vi "host 1st.vi"() -> ()   [LabVIEW 2017]
uses:
  b7b9a1d8-5f4e-4797-a25c-3bdebfd9df9c.vi
  globals/Global variables.vi
  globals/RIO and DAC defaults global.vi
  globals/Modules global.vi
  globals/DIO board parameters global.vi
  <vilib>/FPGAPlugInAG/PXI-7811R/niLvFpga_Open_PXI-7811R.vi
  <vilib>/rvi/interface/common/dynamic/niFpgaDynamicAddResources.vi
  <vilib>/rvi/interface/nirviOpenFPGA/nirviOpenFPGA.xnode
  FPGA Bitfiles/project1_FPGATarget_statemachine_BoC7x3TXtqU.lvbitx
  FPGA vi/state machine.vi
panel:
  out "GPIB output":T1(array[cluster])=[{"Enable"=TRUE, "Abs Start Time"=26343.857, "Module"=31, "String"="FREQ 2 MHz;", "Array"=["27", ""]}, {"Enable"=TRUE, "Abs Start Time"=27143.857, "Module"=31, "String"="ENBR 1;", "Array"=["27", ""]}, {"Enable"=TRUE, "Abs Start Time"=29143.857, "Module"=31, "String"="ENBR 0;", "Array"=["27", ""]}]
  out "AO indicator 3":dbl[][](array[numeric])
  in  "DAC timeline enables 3":bool[](array[boolean])=[FALSE, FALSE, FALSE, FALSE, FALSE, FALSE, FALSE, TRUE]
  out "DAC timelines 3":T2(graph)=[{"times"=[], "Static DAC Array"=[]}, {"times"=[], "Static DAC Array"=[]}, {"times"=[], "Static DAC Array"=[]}, {"times"=[], "Static DAC Array"=[]}, {"times"=[], "Static DAC Array"=[]}, {"times"=[], "Static DAC Array"=[]}, {"times"=[], "Static DAC Array"=[]}, {"times"=[0.1, 1501.0, 1501.1, 1501.2, 1501.3, 1501.4, 1501.5, 1501.6, 1501.7, 1501.8, 1501.9, 1502.0, 1600.0, 1700.0, 1800.0, 8000.0], "Static DAC Array"=[0.0, 0.0, 0.5, 1.0, 1.5, 2.0, 2.5, 3.0, 3.5, 4.0, 4.5, 5.0, 1.0, 2.0, 3.0, 0.0]}]
  in  "DAC force enables 3":bool[](array[boolean])=[FALSE, FALSE, FALSE, FALSE, FALSE, FALSE, FALSE, FALSE]
  in  "DAC force volts 3":dbl[](array[numeric])=[0.0, 0.0, 0.0, 0.0, 0.0, 0.0, 0.0, 0.0]
  out "DAC channel discription 3":string[](array[string])=["", "", "", "", "", "", "", "\n"]
  out "number 2":ext=24208.27054977417 format="%#_9g"
  out "number":ext=2000.0 format="%#_9g"
  out "Boolean 6":bool
  out "Boolean 5":bool
  out "Boolean 4":bool
  out "Boolean 3":bool
  out "Boolean 2":bool
  out "Boolean":bool
  out "millisecond timer value 6":u32=8013
  out "millisecond timer value 5":u32=24245
  out "millisecond timer value 4":u32=2034
  out "millisecond timer value 3":u32=34
  out "millisecond timer value 2":u32=34
  in  "Load commands":bool
  in  "Save commands":bool
  out "Command picked":string="Run experiment for 4 cycles, CODE "
  out "AO indicator 2":dbl[][](array[numeric])
  out "AO indicator 1":dbl[][](array[numeric])=[[0.0, 0.0, 0.0, 3.0, 0.0, 0.0, 0.0, 0.0], [0.0, 0.0, 0.0, 3.0, 0.0, 0.0, 0.0, 0.0]]
  out "DO port C/D indicator":u64[](array[numeric])
  out "DO port A/B indicator":u64[](array[numeric])=[562949970739728, 562949970739728]
  out "DO timing indicator":u64[](array[numeric])=[0, 34142857]
  in  "Clear Error":bool
  out "timing check":dbl=6.484375 format="%.3f"
  out "time 2":dbl=0.03800153732299805
  out "t_start":dbl=3608872841.2628255
  out "temp command":string
  out "FPGA Error":errorcluster
  in  "Check timing?":bool
  in  "Run single shot":bool
  in  "Run programmed\ndata acquisition":bool
  out "Error message":string="Done."
  out "Max module time":dbl=8000.0
  in  "Section enables":bool[](array[boolean])=[TRUE, TRUE, TRUE, TRUE, TRUE, TRUE, TRUE]
  in  "Load backup?":bool
  in  "Stop Experiment":bool
  out "Command window":string="Run experiment for 4 cycles, CODE 05\n\n"
  in  "Enable programming\n measurement":bool
  in  "Tree for programmed measurement":string(tree)="Run N cycles"
  in  "Modules\nDo write/read":bool
  in  "Write/read modules":bool
  in  "Modules save file name":string="testing"
  in  "Sequence\nDo write/read":bool
  in  "Write/read\nmodule sequence":bool
  in  "Select module sequence":u16(ring) items=["MOT recapture", "Most recent expt", "Quadrupole trap", "MOT fill", "BEC", "FORT with transfers", "ZP beam align", "Test1", "Test2", "Align probe beam", "Test3", "Test4", "Test5", "Blank", "Roundtrip MOT recapture", "IP trap load recapture"]
  out "Good to go":bool=TRUE
  in  "Open module":bool
  in  "Select module":u16(ring)=34 items=["Atom removal 1", "Atom removal 2", "B-field off", "CMOT", "Defaults", "Final B-field ramps", "Fluorescence pulse", "High field", "High field ARP", "Loading cart QT", "Loading sci QT", "Low field", "Low field ARP", "Mol OD image", "Mol picture", "Mol probe pulse", "Molasses", "MOT off", "MOT on", "OD image", "Optical pumping", "OT B-field off", "Picture", "Probe pulse", "QT off for OT", "Quadrupole trap off", "Quadrupole trap", "Quantization axis", "S-G separation", "STIRAP back for imaging", "STIRAP", "TTL high", "TTL low", "GPIB", "Utility Module 1", "Utility Module 2", "Utility Module 3", "Utility Module 4", "Utility Module 5", "Utility Module 6", "Utility Module 7", "Utility Module 8", "Utility Module 9"]
  in  "DAC timeline enables 2":bool[](array[boolean])=[FALSE, FALSE, FALSE, FALSE, FALSE, FALSE, FALSE, FALSE]
  in  "DAC timeline enables 1":bool[](array[boolean])=[FALSE, FALSE, FALSE, FALSE, FALSE, FALSE, FALSE, FALSE]
  out "DAC timelines 2":T2(graph)
  out "DAC timelines 1":T2(graph)
  out "RIO timelines":cluster{u32[], i32[]}[](graph)
  in  "RIO timeline enables":bool[][](array[boolean])
  in  "DAC defaults":bool
  in  "Force DAC outputs":bool
  out "DAC channel discription 2":string[](array[string])=["", "", "", "", "", "", "", "\n"]
  out "DAC channel discription 1":string[](array[string])=["aaa", "", "", "", "", "", "", " \n"]
  in  "DAC force volts 2":dbl[](array[numeric])=[0.0, 0.0, 0.0, 0.0, 0.0, 0.0, 0.0, 0.0]
  in  "DAC force volts 1":dbl[](array[numeric])=[0.0, 0.0, 0.0, 3.0, 0.0, 0.0, 0.0, 0.0]
  in  "DAC force enables 2":bool[](array[boolean])=[FALSE, FALSE, FALSE, FALSE, FALSE, FALSE, FALSE, FALSE]
  in  "DAC force enables 1":bool[](array[boolean])=[FALSE, TRUE, FALSE, FALSE, FALSE, FALSE, FALSE, TRUE]
  in  "RIO defaults":bool
  in  "Force RIO outputs":bool
  in  "Port D forced outputs":bool[](array[boolean])=[FALSE, FALSE, FALSE, FALSE, FALSE, FALSE, FALSE, FALSE, FALSE, FALSE, FALSE, FALSE, FALSE, FALSE, FALSE, FALSE, FALSE, FALSE, FALSE, FALSE, FALSE, FALSE, FALSE, FALSE, FALSE, FALSE, FALSE, FALSE, FALSE, FALSE, FALSE, FALSE]
  in  "Port C forced outputs":bool[](array[boolean])=[FALSE, FALSE, FALSE, FALSE, FALSE, FALSE, FALSE, FALSE, FALSE, FALSE, FALSE, FALSE, FALSE, FALSE, FALSE, FALSE, FALSE, FALSE, FALSE, FALSE, FALSE, FALSE, FALSE, FALSE, FALSE, FALSE, FALSE, FALSE, FALSE, FALSE, FALSE, FALSE]
  in  "Port B forced outputs":bool[](array[boolean])=[FALSE, FALSE, FALSE, FALSE, FALSE, FALSE, FALSE, FALSE, FALSE, FALSE, FALSE, FALSE, FALSE, FALSE, FALSE, FALSE, FALSE, TRUE, FALSE, FALSE, FALSE, FALSE, FALSE, FALSE, FALSE, FALSE, FALSE, FALSE, FALSE, FALSE, FALSE, FALSE]
  in  "Port A forced outputs":bool[](array[boolean])=[FALSE, FALSE, FALSE, FALSE, TRUE, FALSE, FALSE, FALSE, FALSE, TRUE, FALSE, FALSE, FALSE, FALSE, TRUE, FALSE, FALSE, FALSE, FALSE, TRUE, FALSE, FALSE, FALSE, FALSE, TRUE, FALSE, FALSE, FALSE, FALSE, FALSE, FALSE, FALSE]
  in  "Durations":string[](array[string])=["1000", "1000", "  1000.000", "1000", "1000", "1000", "1000"]
  in  "Tab Control":T3(tab)=enum."After opt trap"
  in  "After MOT fill comments":string="Comment Here:"
  in  "Modules 1":T4(array[cluster])=[{"enable"=FALSE, "start time"="500", "module"=34, "comment and discription"="", "Port and line"=[]}] {"module" items=["Atom removal 1", "Atom removal 2", "B-field off", "CMOT", "Defaults", "Final B-field ramps", "Fluorescence pulse", "High field", "High field ARP", "Loading cart QT", "Loading sci QT", "Low field", "Low field ARP", "Mol OD image", "Mol picture", "Mol probe pulse", "Molasses", "MOT off", "MOT on", "OD image", "Optical pumping", "OT B-field off", "Picture", "Probe pulse", "QT off for OT", "Quadrupole trap off", "Quadrupole trap", "Quantization axis", "S-G separation", "STIRAP back for imaging", "STIRAP", "TTL high", "TTL low", "GPIB", "Utility Module 1", "Utility Module 2", "Utility Module 3", "Utility Module 4", "Utility Module 5", "Utility Module 6", "Utility Module 7", "Utility Module 8", "Utility Module 9"]}
  in  "After hold comments":string="Comment Here:"
  in  "Modules 2":T4(array[cluster])=[{"enable"=FALSE, "start time"="0", "module"=0, "comment and discription"="", "Port and line"=[]}] {"module" items=["Atom removal 1", "Atom removal 2", "B-field off", "CMOT", "Defaults", "Final B-field ramps", "Fluorescence pulse", "High field", "High field ARP", "Loading cart QT", "Loading sci QT", "Low field", "Low field ARP", "Mol OD image", "Mol picture", "Mol probe pulse", "Molasses", "MOT off", "MOT on", "OD image", "Optical pumping", "OT B-field off", "Picture", "Probe pulse", "QT off for OT", "Quadrupole trap off", "Quadrupole trap", "Quantization axis", "S-G separation", "STIRAP back for imaging", "STIRAP", "TTL high", "TTL low", "GPIB", "Utility Module 1", "Utility Module 2", "Utility Module 3", "Utility Module 4", "Utility Module 5", "Utility Module 6", "Utility Module 7", "Utility Module 8", "Utility Module 9"]}
  in  "Evaporation comments":string="Comment Here:"
  in  "Do Evap":bool
  in  "Sweeps":T5(array[cluster])=[{"Enable MW"=FALSE, "MW End freq"="6810", "MW Tau (s)"="7", "MW Amplitude (dB)"="-3", "MW Comments"=""}, {"Enable MW"=FALSE, "MW End freq"="6820", "MW Tau (s)"="7", "MW Amplitude (dB)"="-5", "MW Comments"=""}, {"Enable MW"=FALSE, "MW End freq"="6830", "MW Tau (s)"="5", "MW Amplitude (dB)"="-5", "MW Comments"=""}, {"Enable MW"=FALSE, "MW End freq"="6832", "MW Tau (s)"="1", "MW Amplitude (dB)"="-7", "MW Comments"=""}, {"Enable MW"=FALSE, "MW End freq"="6833.22", "MW Tau (s)"="1", "MW Amplitude (dB)"="-8", "MW Comments"=""}]
  in  "Start freq (MHz)":string="6700.00"
  in  "Ramp start time (s)":string="1.000"
  out "Calc'd time":dbl=1.0
  in  "Modules 3":T4(array[cluster])=[{"enable"=FALSE, "start time"="0", "module"=0, "comment and discription"="", "Port and line"=[]}] {"module" items=["Atom removal 1", "Atom removal 2", "B-field off", "CMOT", "Defaults", "Final B-field ramps", "Fluorescence pulse", "High field", "High field ARP", "Loading cart QT", "Loading sci QT", "Low field", "Low field ARP", "Mol OD image", "Mol picture", "Mol probe pulse", "Molasses", "MOT off", "MOT on", "OD image", "Optical pumping", "OT B-field off", "Picture", "Probe pulse", "QT off for OT", "Quadrupole trap off", "Quadrupole trap", "Quantization axis", "S-G separation", "STIRAP back for imaging", "STIRAP", "TTL high", "TTL low", "GPIB", "Utility Module 1", "Utility Module 2", "Utility Module 3", "Utility Module 4", "Utility Module 5", "Utility Module 6", "Utility Module 7", "Utility Module 8", "Utility Module 9"]}
  in  "After evap comments":string="Comment Here:"
  in  "After mag trap comments":string="Comment Here:"
  in  "Modules 4":T4(array[cluster])=[{"enable"=FALSE, "start time"="0", "module"=0, "comment and discription"="", "Port and line"=[]}] {"module" items=["Atom removal 1", "Atom removal 2", "B-field off", "CMOT", "Defaults", "Final B-field ramps", "Fluorescence pulse", "High field", "High field ARP", "Loading cart QT", "Loading sci QT", "Low field", "Low field ARP", "Mol OD image", "Mol picture", "Mol probe pulse", "Molasses", "MOT off", "MOT on", "OD image", "Optical pumping", "OT B-field off", "Picture", "Probe pulse", "QT off for OT", "Quadrupole trap off", "Quadrupole trap", "Quantization axis", "S-G separation", "STIRAP back for imaging", "STIRAP", "TTL high", "TTL low", "GPIB", "Utility Module 1", "Utility Module 2", "Utility Module 3", "Utility Module 4", "Utility Module 5", "Utility Module 6", "Utility Module 7", "Utility Module 8", "Utility Module 9"]}
  in  "After opt trap comments":string="Comment Here:"
  in  "Modules 5":T4(array[cluster])=[{"enable"=TRUE, "start time"="1", "module"=34, "comment and discription"="", "Port and line"=[]}] {"module" items=["Atom removal 1", "Atom removal 2", "B-field off", "CMOT", "Defaults", "Final B-field ramps", "Fluorescence pulse", "High field", "High field ARP", "Loading cart QT", "Loading sci QT", "Low field", "Low field ARP", "Mol OD image", "Mol picture", "Mol probe pulse", "Molasses", "MOT off", "MOT on", "OD image", "Optical pumping", "OT B-field off", "Picture", "Probe pulse", "QT off for OT", "Quadrupole trap off", "Quadrupole trap", "Quantization axis", "S-G separation", "STIRAP back for imaging", "STIRAP", "TTL high", "TTL low", "GPIB", "Utility Module 1", "Utility Module 2", "Utility Module 3", "Utility Module 4", "Utility Module 5", "Utility Module 6", "Utility Module 7", "Utility Module 8", "Utility Module 9"]}
  in  "New stuff comments":string="Comment Here:"
  in  "Modules 6":T4(array[cluster])=[{"enable"=TRUE, "start time"="2000", "module"=4, "comment and discription"="", "Port and line"=[]}, {"enable"=FALSE, "start time"="", "module"=0, "comment and discription"="", "Port and line"=[]}] {"module" items=["Atom removal 1", "Atom removal 2", "B-field off", "CMOT", "Defaults", "Final B-field ramps", "Fluorescence pulse", "High field", "High field ARP", "Loading cart QT", "Loading sci QT", "Low field", "Low field ARP", "Mol OD image", "Mol picture", "Mol probe pulse", "Molasses", "MOT off", "MOT on", "OD image", "Optical pumping", "OT B-field off", "Picture", "Probe pulse", "QT off for OT", "Quadrupole trap off", "Quadrupole trap", "Quantization axis", "S-G separation", "STIRAP back for imaging", "STIRAP", "TTL high", "TTL low", "GPIB", "Utility Module 1", "Utility Module 2", "Utility Module 3", "Utility Module 4", "Utility Module 5", "Utility Module 6", "Utility Module 7", "Utility Module 8", "Utility Module 9"]}
  # "0     1     2     3     4     5     6     7     8     9    10   11   12   13   14   15   16   17   18   19   20   21   22   23   24   25   26   27   28   29   30   31"
  # "Indicators for debugging"
  # "A"
  # "B"
  # "C"
  # "Read"
  # "Write"
  # "D"
  # "MOT fill (ms)"
  # "Hold"
  # "Evaporation"
  # "Magnetic trap"
  # "Optical trap"
  # "New"
  # "Read"
  # "Write"
  # "Volts"
  # "Description"
  # "0"
  # "1"
  # "2"
  # "3"
  # "4"
  # "5"
  # "6"
  # "7"
  # "8"
  # "9"
  # "10"
  # "11"
  # "12"
  # "13"
  # "14"
  # "15"
  # "16"
  # "17"
  # "18"
  # "19"
  # "20"
  # "21"
  # "22"
  # "23"
  # "After MOT fill"
  # "Enable     Time                        Module                           Port     Line                  Comments                                                        \n                                                                                         (A~D)  (0~31)"
  # "After hold"
  # "Enable     Time                        Module                           Port     Line                  Comments                                                        \n                                                                                         (A~D)  (0~31)"
  # "Evaporation"
  # "tau (s)"
  # "amplitude (s)"
  # "comments"
  # "enable"
  # "end freq (MHz)"
  # "After evaporation"
  # "Enable     Time                        Module                           Port     Line                  Comments                                                        \n                                                                                         (A~D)  (0~31)"
  # "After magnetic trap"
  # "Enable     Time                        Module                           Port     Line                  Comments                                                        \n                                                                                         (A~D)  (0~31)"
  # "After optical trap"
  # "Enable     Time                        Module                           Port     Line                  Comments                                                        \n                                                                                         (A~D)  (0~31)"
  # "New stuff"
  # "Enable     Time                        Module                           Port     Line                  Comments                                                        \n                                                                                         (A~D)  (0~31)"
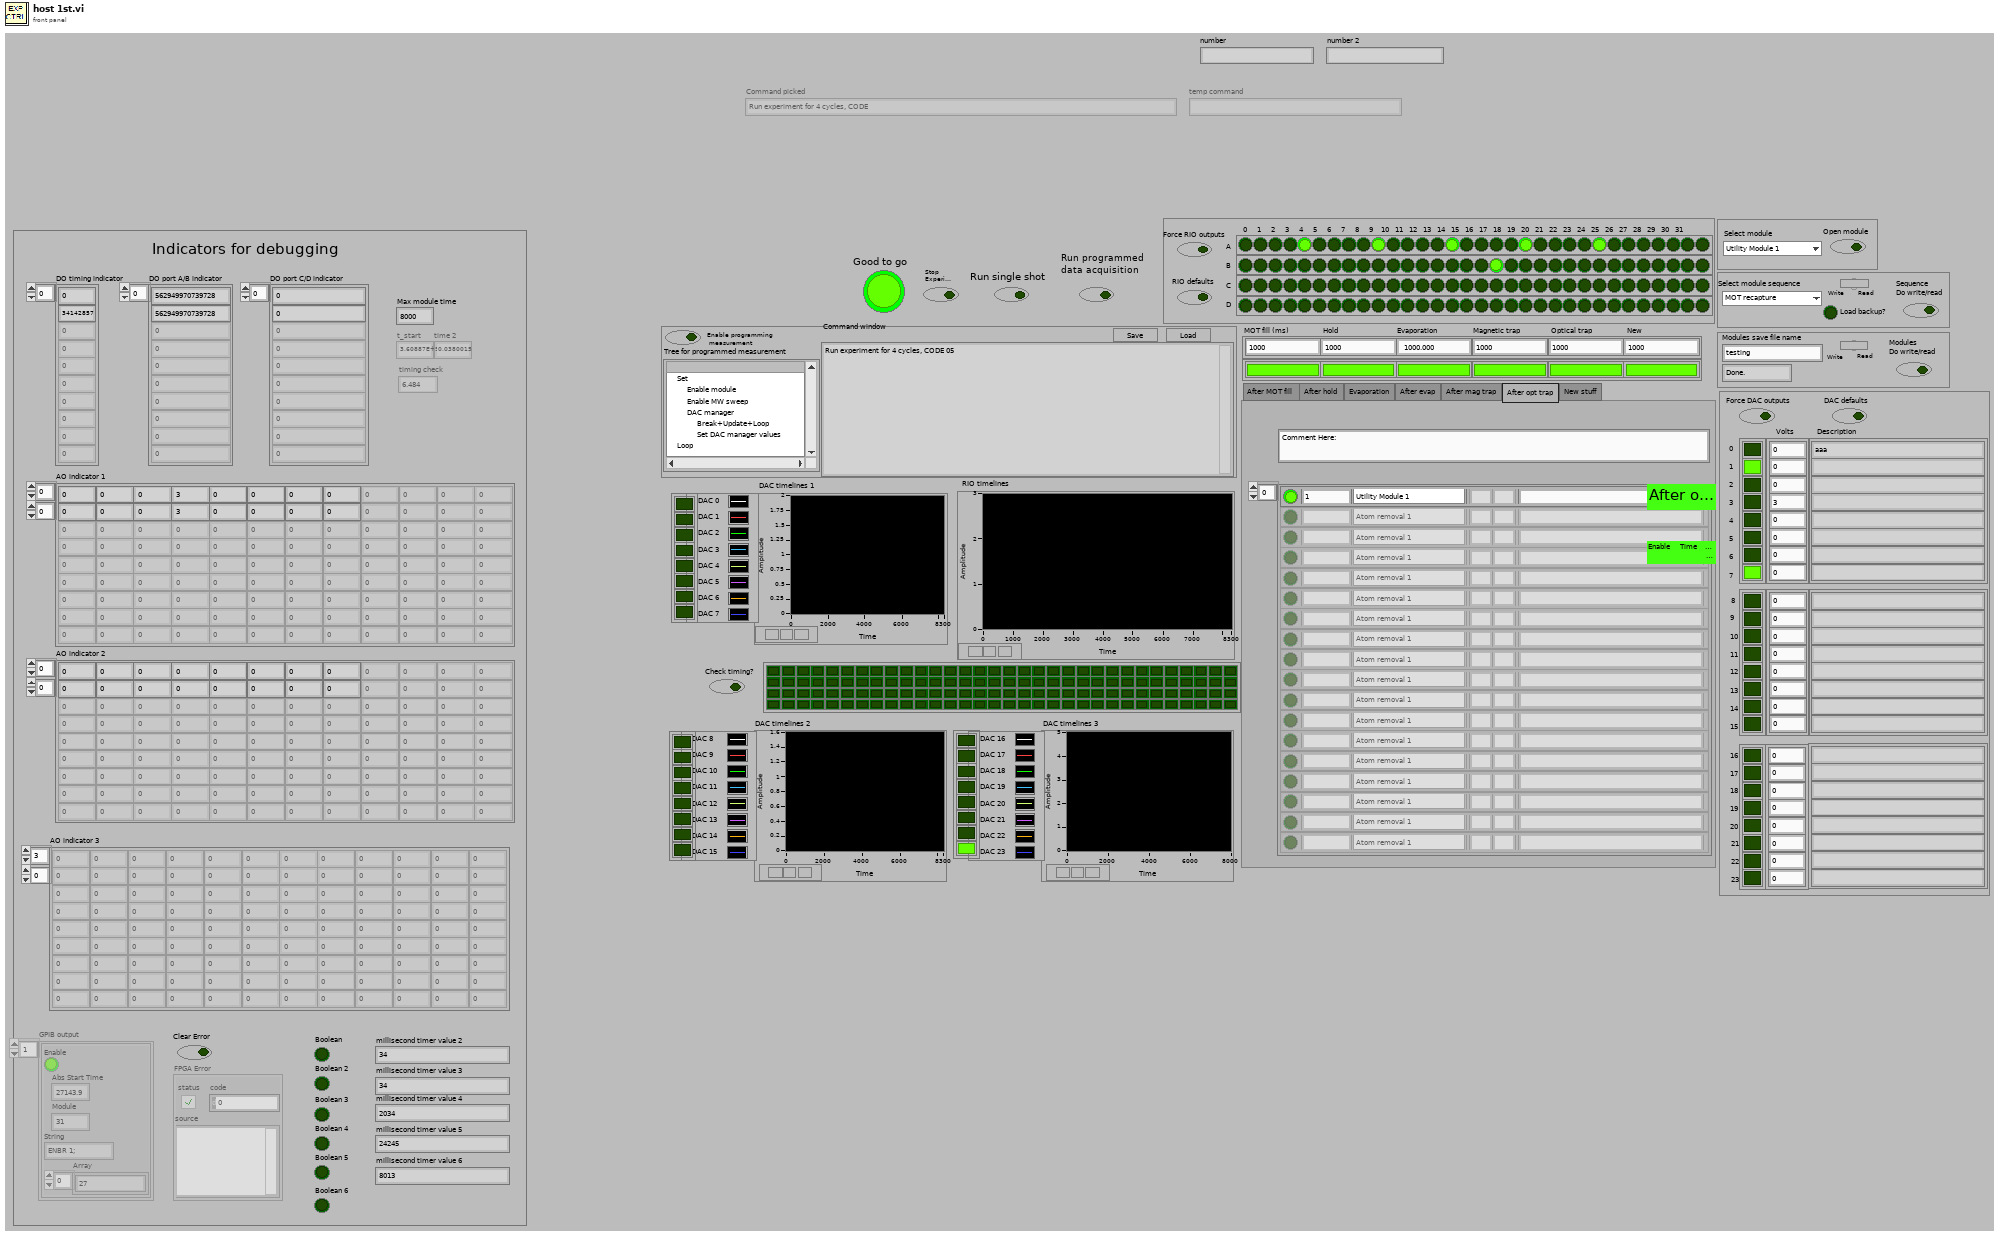
[diagram p1: front panel]
types:
  T1 = cluster{"Enable":bool, "Abs Start Time":dbl, "Module":u16, "String":string, "Array":string[]}[]
  T2 = cluster{"times":dbl[], "Static DAC Array":dbl[]}[]
  T3 = enum32{"After MOT fill", "After hold", "Evaporation", "After evap", "After mag trap", "After opt trap", "New stuff"}
  T4 = cluster{"enable":bool, "start time":string, "module":u16, "comment and discription":string, "Port and line":string[]}[]
  T5 = cluster{"Enable MW":bool, "MW End freq":string, "MW Tau (s)":string, "MW Amplitude (dB)":string, "MW Comments":string}[]
  T6 = enum8{"Enabled", "Disabled", "Disabled and Grayed Out"}
  T7 = cluster{"Modules 1":cluster{"enable":bool, "start time":string, "module":u16, "comment and discription":string, "Port and line":string[]}[], "Modules 2":cluster{"enable":bool, "start time":string, "module":u16, "comment and discription":string, "Port and line":string[]}[], "Modules 3":cluster{"enable":bool, "start time":string, "module":u16, "comment and discription":string, "Port and line":string[]}[], "Modules 4":cluster{"enable":bool, "start time":string, "module":u16, "comment and discription":string, "Port and line":string[]}[], "Modules 5":cluster{"enable":bool, "start time":string, "module":u16, "comment and discription":string, "Port and line":string[]}[], "Modules 6":cluster{"enable":bool, "start time":string, "module":u16, "comment and discription":string, "Port and line":string[]}[]}
  T8 = cluster{"Ramp start time (s)":string, "Start freq (MHz)":string, "Sweeps":cluster{"Enable MW":bool, "MW End freq":string, "MW Tau (s)":string, "MW Amplitude (dB)":string, "MW Comments":string}[]}
  T9 = cluster{cluster{"Modules 1":cluster{"enable":bool, "start time":string, "module":u16, "comment and discription":string, "Port and line":string[]}[], "Modules 2":cluster{"enable":bool, "start time":string, "module":u16, "comment and discription":string, "Port and line":string[]}[], "Modules 3":cluster{"enable":bool, "start time":string, "module":u16, "comment and discription":string, "Port and line":string[]}[], "Modules 4":cluster{"enable":bool, "start time":string, "module":u16, "comment and discription":string, "Port and line":string[]}[], "Modules 5":cluster{"enable":bool, "start time":string, "module":u16, "comment and discription":string, "Port and line":string[]}[], "Modules 6":cluster{"enable":bool, "start time":string, "module":u16, "comment and discription":string, "Port and line":string[]}[]}, "Durations":string[], cluster{"Ramp start time (s)":string, "Start freq (MHz)":string, "Sweeps":cluster{"Enable MW":bool, "MW End freq":string, "MW Tau (s)":string, "MW Amplitude (dB)":string, "MW Comments":string}[]}}
  T10 = cluster{cluster{"Module List 1":cluster{"Enable":bool, "Abs Start Time":string, "Module":u16, "String":string, "Array":string[]}[], "Module List 2":cluster{"Enable":bool, "Abs Start Time":string, "Module":u16, "String":string, "Array":string[]}[], "Module List 3":cluster{"Enable":bool, "Abs Start Time":string, "Module":u16, "String":string, "Array":string[]}[], "Module List 4":cluster{"Enable":bool, "Abs Start Time":string, "Module":u16, "String":string, "Array":string[]}[], "Module List 5":cluster{"Enable":bool, "Abs Start Time":string, "Module":u16, "String":string, "Array":string[]}[], "Module List 6":cluster{"Enable":bool, "Abs Start Time":string, "Module":u16, "String":string, "Array":string[]}[]}, string[], "evap cluster":cluster{"Start Freq (MHz)":string, "Ramp Start Time (s)":string, "Sweeps":cluster{"Enable":bool, "Freq (MHz)":string, "Tau (s)":string, "Amp (dBm)":string, "Notes":string}[]}}
  T11 = cluster{"Module List 1":cluster{"Enable":bool, "Abs Start Time":string, "Module":u16, "String":string, "Array":string[]}[], "Module List 2":cluster{"Enable":bool, "Abs Start Time":string, "Module":u16, "String":string, "Array":string[]}[], "Module List 3":cluster{"Enable":bool, "Abs Start Time":string, "Module":u16, "String":string, "Array":string[]}[], "Module List 4":cluster{"Enable":bool, "Abs Start Time":string, "Module":u16, "String":string, "Array":string[]}[], "Module List 5":cluster{"Enable":bool, "Abs Start Time":string, "Module":u16, "String":string, "Array":string[]}[], "Module List 6":cluster{"Enable":bool, "Abs Start Time":string, "Module":u16, "String":string, "Array":string[]}[]}
  T12 = cluster{"Start Freq (MHz)":string, "Ramp Start Time (s)":string, "Sweeps":cluster{"Enable":bool, "Freq (MHz)":string, "Tau (s)":string, "Amp (dBm)":string, "Notes":string}[]}
  T13 = cluster{"Enable":bool, "Freq (MHz)":string, "Tau (s)":string, "Amp (dBm)":string, "Notes":string}[]
  T14 = cluster{"Enable":bool, "Abs Start Time":string, "Module":u16, "String":string, "Array":string[]}[]
  T15 = cluster{"Enable MW":bool, "MW End freq":string, "MW Tau (s)":string, "MW Amplitude (dB)":string, "MW Comments":string}
  T16 = cluster{"enable":bool, "start time":string, "module":u16, "comment and discription":string, "Port and line":string[]}
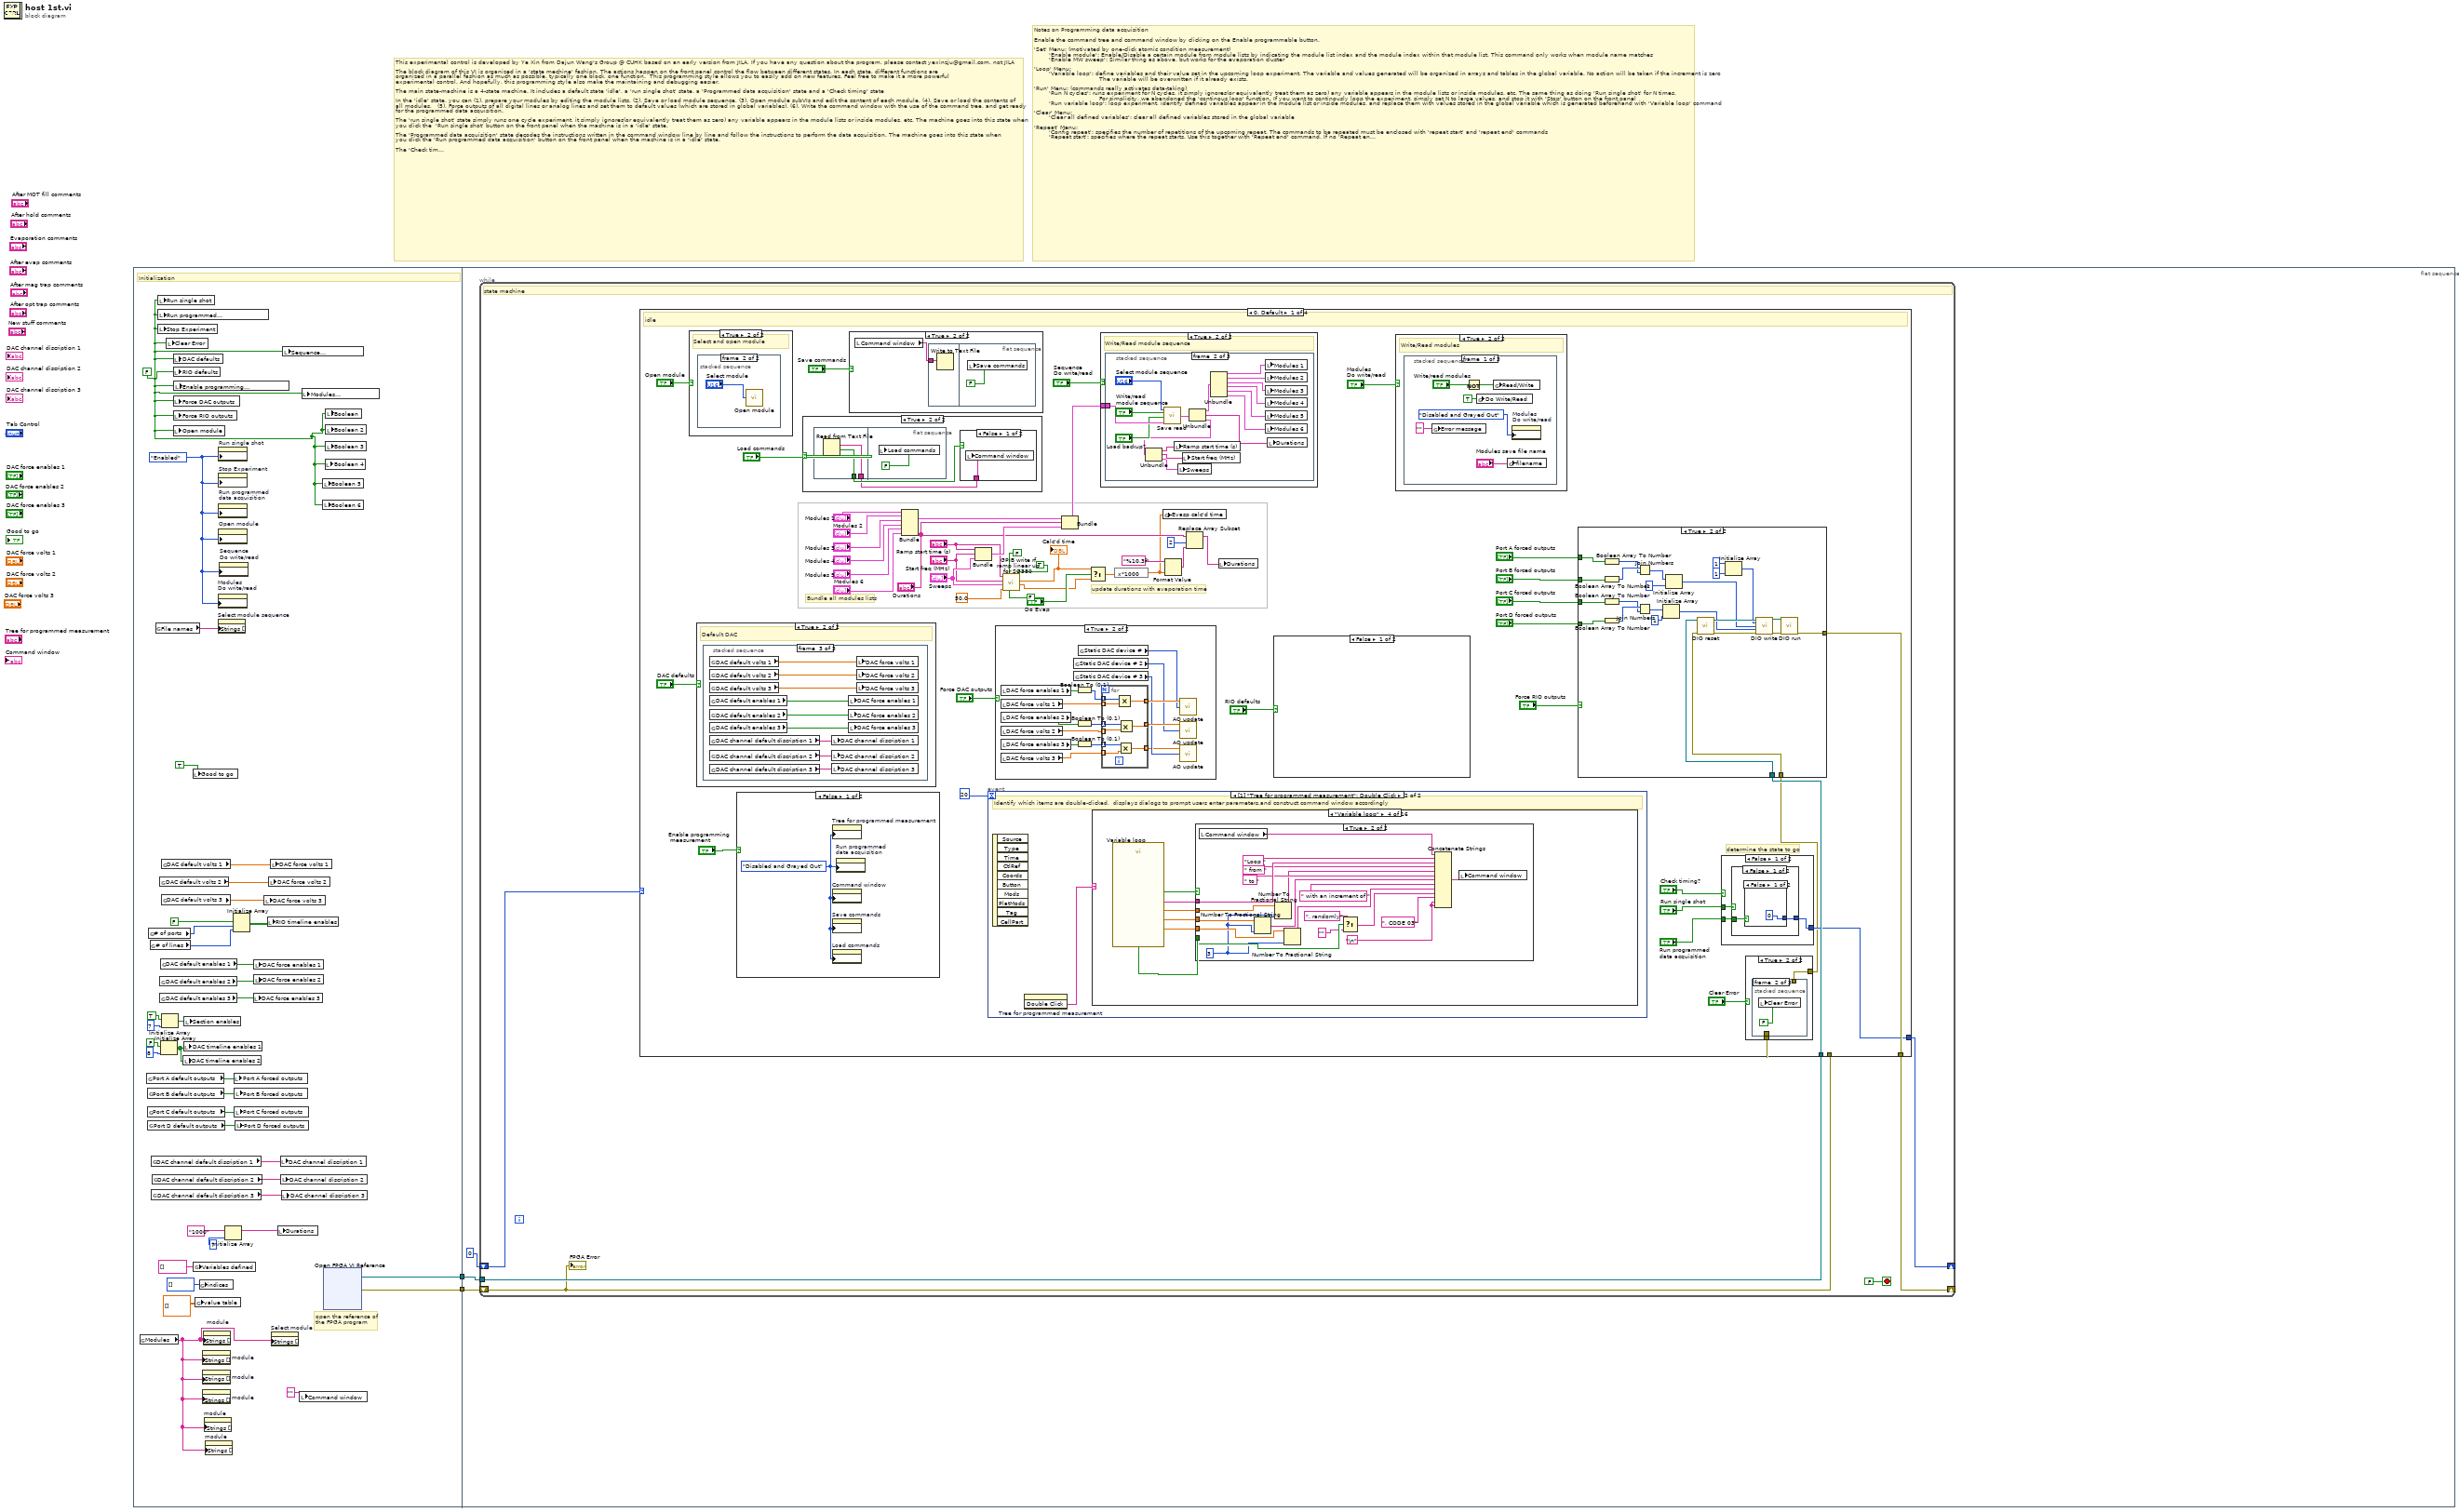
[diagram p0: block diagram]
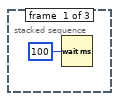
[diagram p6: hidden frame]
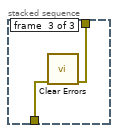
[diagram p7: hidden frame]
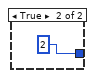
[diagram p8: hidden frame]
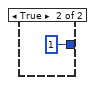
[diagram p9: hidden frame]
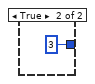
[diagram p10: hidden frame]
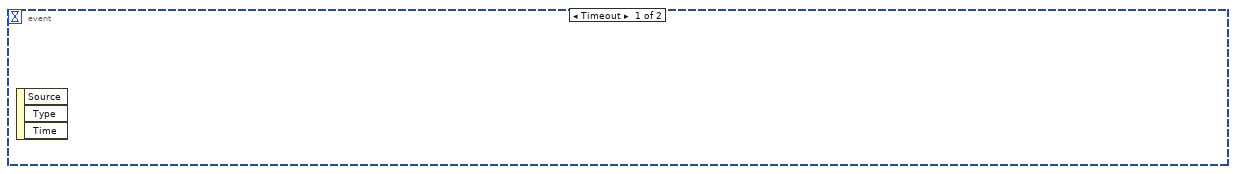
[diagram p11: hidden frame]
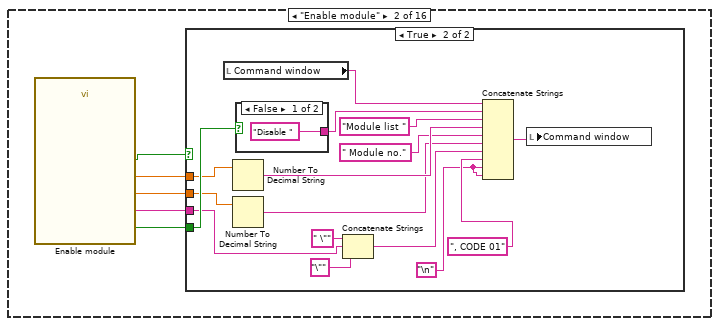
[diagram p13: hidden frame]
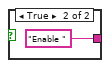
[diagram p15: hidden frame]
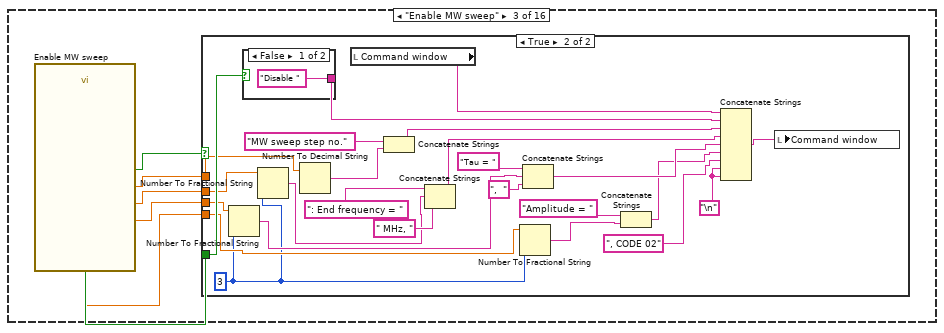
[diagram p16: hidden frame]
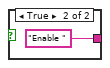
[diagram p18: hidden frame]
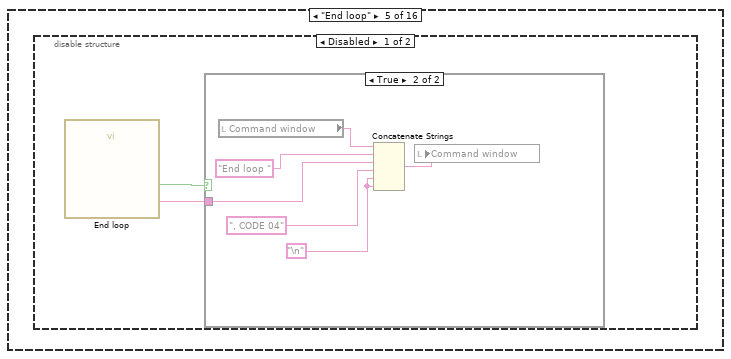
[diagram p20: hidden frame]
diagram:
  # "Notes on Programming data acquisition\n\nEnable the command tree and command window by clicking on the Enable programmable button.\n\n'Set' Menu: (motivated by one-click atomic condition measurement)\n        'Enable module': Enable/Disable a certain module from module lists by indicating the module list index and the module index within that module list. This command only works when module name matches\n        'Enable MW sweep': Similar thing as above, but works for the evaporation cluster\n\n'Loop' Menu:\n        'Variable loop': define variables and their value set in the upcoming loop experiment. The variable and values generated will be organized in arrays and tables in the global variable. No action will be taken if the increment is zero\n                                   The variable will be overwritten if it already exists.\n\n'Run' Menu: (commands really activates data-taking)\n        'Run N cycles': runs experiment for N cycles, it simply ignores(or equivalently treat them as zero) any variable appears in the module lists or inside modules, etc. The same thing as doing 'Run single shot' for N times.\n                                   For simplicity, we abandoned the 'continous loop' function. If you want to continously loop the experiment, simply set N to large values, and stop it with 'Stop' button on the front panel\n        'Run variable loop': loop experiment, identify defined variables appear in the module list or inside modules, and replace them with values stored in the global variable which is generated beforehand with 'Variable loop' command\n\n'Clear' Menu:\n        'Clear all defined variables': clear all defined variables stored in the global variable\n\n'Repeat' Menu:\n        'Config repeat': specifies the number of repetitions of the upcoming repeat. The commands to be repeated must be enclosed with 'repeat start' and 'repeat end' commands\n        'Repeat start': specifies where the repeat starts. Use this together with 'Repeat end' command. If no 'Repeat end' comes after 'Repeat start', all commands till the end will be repeated. But this practice is strongly not recommended\n        'Repeat end': specifies where the repeat ends, Use this together with 'Repeat start' command. If no' Repeat start' appears before 'Repeat end', nothing happens. But this practice is strongly not recommended\n\n'Edit' Menu: (provide standard ways to modify the content of the command window, reduce the possibility of error by manually modifying it with cursor)\n        'Move': advance or defer certain command already exists in the command window\n        'Swap': swap the positions of two commands in the command window\n        'Delete': delete a certain command or all commands from the command window"
  # "This experimental control is developed by Ye Xin from Dajun Wang's Group @ CUHK based on an early version from JILA. If you have any question about the program, please contact yexinzju@gmail.com, not JILA\n\nThe block diagram of this VI is organized in a 'state mechine' fashion. The actions happen on the front panel control the flow between different states. In each state, different functions are \norganized in a parallel fashion as much as possible, typically one block, one function.  This programming style allows you to easily add on new features. Feel free to make it a more powerful\nexperimental control. And hopefully, this programming style also make the maintaining and debugging easier.\n\nThe main state-machine is a 4-state machine. It includes a default state 'idle', a 'run single shot' state, a 'Programmed data acquisition' state and a 'Check timing' state\n\nIn the 'idle' state, you can (1). prepare your modules by editing the module lists, (2). Save or load module sequence, (3). Open module subVIs and edit the content of each module, (4). Save or load the contents of \nall modules,   (5). Force outputs of all digital lines or analog lines and set them to default values (which are stored in global variables), (6). Write the command window with the use of the command tree, and get ready\nfor the programmed data acquisition.\n\nThe 'run single shot' state simply runs one cycle experiment, it simply ignores(or equivalently treat them as zero) any variable appears in the module lists or inside modules, etc. The machine goes into this state when\nyou click the  'Run single shot' button on the front panel when the machine is in a 'idle' state. \n\nThe 'Programmed data acquisition' state decodes the instructions written in the command window line by line and follow the instructions to perform the data acquisition. The machine goes into this state when\nyou click the 'Run programmed data acquisition' button on the front panel when the machine is in a 'idle' state.\n\nThe 'Check timing' state returns you three diagrams on the front panel to show the timings and outputs of all lines with your current settings. The machine goes into this state whenyou click the 'Check timing?' button \non the front panel when the machine is in a 'idle' state.\n\nWhen the machine finishes tasks or button 'Stop' is clicked on during 'Programmed data acquisition' state, it always returns back to the 'idle' state.\n\nThe current control is originally designed for 'NI PXI-7811R', 'NI PXI-6713' and 'NI PXI-6733', but things should be quite universal for hardwares within the NI family. Not many changes should be made if you swith to other \nhardwares. The changes may depend on the total channel number, clock frequency etc."
  n1 = flat-sequence {
    tunnel: [w7] -> w2
    tunnel: [w6] -> w1
    tunnel: w2 -> [w42]
    tunnel: w1 -> [w41]
    frame #0 {
      w11 = T6."Enabled" ("Disabled")
      w8 = FALSE ("Abort")
      # "open the reference of\nthe FPGA program"
      # "Initialization"
      n2 = global read "Modules global.vi" "Modules"() -> (w16:string[])
      n3 = global read "RIO and DAC defaults global.vi" "Port A default outputs"() -> (w35:bool[])
      n4 = global read "RIO and DAC defaults global.vi" "Port B default outputs"() -> (w36:bool[])
      n5 = global read "RIO and DAC defaults global.vi" "Port C default outputs"() -> (w34:bool[])
      n6 = global read "RIO and DAC defaults global.vi" "Port D default outputs"() -> (w33:bool[])
      n7 = global read "DIO board parameters global.vi" "# of ports"() -> (w10:u16)
      n8 = global read "DIO board parameters global.vi" "# of lines"() -> (w9:u16)
      n9 = global read "RIO and DAC defaults global.vi" "DAC channel default discription 1"() -> (w32:string[])
      n10 = global read "RIO and DAC defaults global.vi" "DAC channel default discription 3"() -> (w3:string[])
      n11 = global read "RIO and DAC defaults global.vi" "DAC channel default discription 2"() -> (w31:string[])
      n12 = global read "Modules global.vi" "File names"() -> (w12:string[])
      n13 = local write "Run single shot"(w8) -> ()
      n14 = local write "Run programmed\ndata acquisition"(w8) -> ()
      n15 = local write "Stop Experiment"(w8) -> ()
      n16 = global read "RIO and DAC defaults global.vi" "DAC default volts 2"() -> (w37:dbl[])
      n17 = global read "RIO and DAC defaults global.vi" "DAC default enables 2"() -> (w14:bool[])
      n18 = global read "RIO and DAC defaults global.vi" "DAC default enables 3"() -> (w4:bool[])
      n19 = global read "RIO and DAC defaults global.vi" "DAC default enables 1"() -> (w13:bool[])
      n20 = Initialize Array(FALSE ("Abort"), 8 ("dimension size")) -> (w20:bool[])
      n21 = global read "RIO and DAC defaults global.vi" "DAC default volts 1"() -> (w38:dbl[])
      n22 = global read "RIO and DAC defaults global.vi" "DAC default volts 3"() -> (w5:dbl[])
      n23 = Initialize Array(TRUE ("Abort"), 7 ("dimension size")) -> (w23:bool[])
      n24 = local write "Clear Error"(w8) -> ()
      n25 = local write "DAC defaults"(w8) -> ()
      n26 = local write "RIO defaults"(w8) -> ()
      n27 = local write "Force DAC outputs"(w8) -> ()
      n28 = local write "Force RIO outputs"(w8) -> ()
      n29 = local write "Open module"(w8) -> ()
      n30 = local write "Enable programming\n measurement"(w8) -> ()
      n31 = local write "DAC timeline enables 2"(w20) -> ()
      n32 = local write "DAC timeline enables 1"(w20) -> ()
      n33 = local write "Section enables"(w23) -> ()
      n34 = local write "Good to go"(TRUE ("Good to go")) -> ()
      n35 = global write "Global variables.vi" "Variables defined"(string[] [] ("Variables defined")) -> ()
      n36 = global write "Global variables.vi" "value table"(dbl[][] [] ("value table")) -> ()
      n37 = global write "Global variables.vi" "indices"(i32[] [] ("indices")) -> ()
      n38 = property on="module" class="Ring (strict)"("Strings []"=w16) -> ()  [unwired: 2 in, 2 out]
      n39 = property on="module" class="Ring (strict)"("Strings []"=w16) -> ()  [unwired: 2 in, 2 out]
      n40 = property on="module" class="Ring (strict)"("Strings []"=w16) -> ()  [unwired: 2 in, 2 out]
      n41 = property on="module" class="Ring (strict)"("Strings []"=w16) -> ()  [unwired: 2 in, 2 out]
      n42 = property on="module" class="Ring (strict)"("Strings []"=w16) -> ()  [unwired: 2 in, 2 out]
      n43 = property on="module" class="Ring (strict)"("Strings []"=w16) -> ()  [unwired: 2 in, 2 out]
      n44 = property on="Modules\nDo write/read" class="Bool (strict)"("DisabledEnum"=w11) -> ()  [unwired: 2 in, 2 out]
      n45 = property on="Select module sequence" class="Ring (strict)"("Strings []"=w12) -> ()  [unwired: 2 in, 2 out]
      n46 = property on="Run single shot" class="Bool (strict)"("DisabledEnum"=w11) -> ()  [unwired: 2 in, 2 out]
      n47 = property on="Stop Experiment" class="Bool (strict)"("DisabledEnum"=w11) -> ()  [unwired: 2 in, 2 out]
      n48 = property on="Run programmed\ndata acquisition" class="Bool (strict)"("DisabledEnum"=w11) -> ()  [unwired: 2 in, 2 out]
      n49 = property on="Open module" class="Bool (strict)"("DisabledEnum"=w11) -> ()  [unwired: 2 in, 2 out]
      n50 = property on="Sequence\nDo write/read" class="Bool (strict)"("DisabledEnum"=w11) -> ()  [unwired: 2 in, 2 out]
      n51 = Initialize Array("1000", 7 ("dimension size")) -> (w26:string[])
      n52 = Initialize Array(FALSE ("Abort"), w10, w9) -> (w29:bool[][])
      n53 = local write "Port A forced outputs"(w35) -> ()
      n54 = local write "Port B forced outputs"(w36) -> ()
      n55 = local write "Port C forced outputs"(w34) -> ()
      n56 = local write "Port D forced outputs"(w33) -> ()
      n57 = local write "DAC force enables 3"(w4) -> ()
      n58 = local write "DAC force enables 1"(w13) -> ()
      n59 = local write "DAC force enables 2"(w14) -> ()
      n60 = local write "DAC force volts 3"(w5) -> ()
      n61 = local write "RIO timeline enables"(w29) -> ()
      n62 = local write "DAC force volts 2"(w37) -> ()
      n63 = local write "DAC force volts 1"(w38) -> ()
      n64 = property on="Select module" class="Ring (strict)"("Strings []"=w16) -> ()  [unwired: 2 in, 2 out]
      n65 = local write "Durations"(w26) -> ()
      n66 = local write "DAC channel discription 1"(w32) -> ()
      n67 = local write "DAC channel discription 2"(w31) -> ()
      n68 = local write "DAC channel discription 3"(w3) -> ()
      n69 = local write "Sequence\nDo write/read"(w8) -> ()
      n70 = local write "Command window"("" ("Command window")) -> ()
      n71 = local write "Modules\nDo write/read"(w8) -> ()
      n72 = local write "Boolean 5"(w8) -> ()
      n73 = local write "Boolean 6"(w8) -> ()
      n74 = xnode "Open FPGA VI Reference"() -> ("FPGA VI Reference Out"=w7:refnum<k20>, "error out"=w6:errorcluster)  [unwired: 2 in]
      n75 = local write "Boolean 4"(w8) -> ()
      n76 = local write "Boolean"(w8) -> ()
      n77 = local write "Boolean 2"(w8) -> ()
      n78 = local write "Boolean 3"(w8) -> ()
    }
    frame #1 {
      n79 = while {
        tunnel: w42 -> [w46]
        shift-right: [w44] -> _
        shift-left: 0 -> [w47]
        shift-right: [w45] -> _
        shift-left: w41 -> [w43]
        stop <- FALSE stop-if-true
        # "state machine"
        n80 = case shown="0, Default" w47 {
          tunnel: w46 -> [w63 w556 w662 _]
          tunnel: w43 -> [w53 w553 w663 w1273]
          tunnel: [w62 w552 w661 w1273] -> w45
          tunnel: [w58 0 0 0] -> w44
          frame 0, Default {
            # "determine the state to go"
            # "update durations with evaporation time"
            # "Bundle all modules lists"
            # "idle"
            n81 = case shown="True" "Open module" {
              frame False {
                # "Pass"
              }
              frame True {
                # "Select and open module"
                n82 = stacked-sequence {
                  frame #0 {
                    n83 = local write "Open module"(FALSE ("Open module")) -> ()
                  }
                  frame #1 {
                    n84 = call "Open module.vi"("Module"="Select module") -> ()
                  }
                }
              }
            }
            n85 = case shown="True" "DAC defaults" {
              frame False {
                # "Pass"
              }
              frame True {
                # "Default DAC"
                n86 = stacked-sequence {
                  frame #0 {
                    n87 = Wait (ms)(milliseconds to wait=u32 100) -> ()  [unwired: 1 out]
                  }
                  frame #1 {
                    n88 = local write "DAC defaults"(FALSE ("RIO defaults")) -> ()
                  }
                  frame #2 {
                    n89 = global read "RIO and DAC defaults global.vi" "DAC default volts 1"() -> (w518:dbl[])
                    n90 = global read "RIO and DAC defaults global.vi" "DAC default volts 2"() -> (w517:dbl[])
                    n91 = global read "RIO and DAC defaults global.vi" "DAC default volts 3"() -> (w512:dbl[])
                    n92 = global read "RIO and DAC defaults global.vi" "DAC default enables 1"() -> (w514:bool[])
                    n93 = global read "RIO and DAC defaults global.vi" "DAC default enables 2"() -> (w513:bool[])
                    n94 = global read "RIO and DAC defaults global.vi" "DAC default enables 3"() -> (w510:bool[])
                    n95 = global read "RIO and DAC defaults global.vi" "DAC channel default discription 1"() -> (w516:string[])
                    n96 = global read "RIO and DAC defaults global.vi" "DAC channel default discription 2"() -> (w515:string[])
                    n97 = global read "RIO and DAC defaults global.vi" "DAC channel default discription 3"() -> (w511:string[])
                    n98 = local write "DAC channel discription 1"(w516) -> ()
                    n99 = local write "DAC channel discription 2"(w515) -> ()
                    n100 = local write "DAC channel discription 3"(w511) -> ()
                    n101 = local write "DAC force enables 1"(w514) -> ()
                    n102 = local write "DAC force enables 2"(w513) -> ()
                    n103 = local write "DAC force enables 3"(w510) -> ()
                    n104 = local write "DAC force volts 1"(w518) -> ()
                    n105 = local write "DAC force volts 2"(w517) -> ()
                    n106 = local write "DAC force volts 3"(w512) -> ()
                  }
                }
              }
            }
            n107 = case shown="False" "Enable programming\n measurement" {
              frame False {
                w451 = T6."Disabled and Grayed Out" ("Disabled")
                n108 = property on="Tree for programmed measurement" class="Tree (strict)"("DisabledEnum"=w451) -> ()  [unwired: 2 in, 2 out]
                n109 = property on="Command window" class="Str"("DisabledEnum"=w451) -> ()  [unwired: 2 in, 2 out]
                n110 = property on="Save commands" class="Bool (strict)"("DisabledEnum"=w451) -> ()  [unwired: 2 in, 2 out]
                n111 = property on="Load commands" class="Bool (strict)"("DisabledEnum"=w451) -> ()  [unwired: 2 in, 2 out]
                n112 = property on="Run programmed\ndata acquisition" class="Bool (strict)"("DisabledEnum"=w451) -> ()  [unwired: 2 in, 2 out]
              }
              frame True {
                w452 = T6."Enabled" ("Disabled")
                n113 = property on="Command window" class="Str"("DisabledEnum"=w452) -> ()  [unwired: 2 in, 2 out]
                n114 = property on="Load commands" class="Bool (strict)"("DisabledEnum"=w452) -> ()  [unwired: 2 in, 2 out]
                n115 = property on="Tree for programmed measurement" class="Tree (strict)"("DisabledEnum"=w452) -> ()  [unwired: 2 in, 2 out]
                n116 = property on="Save commands" class="Bool (strict)"("DisabledEnum"=w452) -> ()  [unwired: 2 in, 2 out]
                n117 = property on="Run programmed\ndata acquisition" class="Bool (strict)"("DisabledEnum"=w452) -> ()  [unwired: 2 in, 2 out]
              }
            }
            n118 = case shown="True" "Load commands" {
              frame False {
              }
              frame True {
                n119 = flat-sequence {
                  tunnel: [w103] -> w99
                  tunnel: [w102] -> w100
                  frame #0 {
                    n120 = Read from Text File() -> (text=w103:string, cancelled=w102:bool)  [unwired: 4 in, 2 out]
                  }
                  frame #1 {
                    n121 = local write "Load commands"(FALSE ("Save commands")) -> ()
                  }
                }
                n122 = case shown="False" w100 {
                  tunnel: w99 -> [w101 _]
                  frame False {
                    n123 = local write "Command window"(w101) -> ()
                  }
                  frame True {
                  }
                }
              }
            }
            n124 = case shown="True" "Save commands" {
              frame False {
              }
              frame True {
                n125 = local read "Command window"() -> (w105:string)
                n126 = flat-sequence {
                  tunnel: w105 -> [w106]
                  frame #0 {
                    n127 = Write to Text File(text=w106) -> ()  [unwired: 3 in, 3 out]
                  }
                  frame #1 {
                    n128 = local write "Save commands"(FALSE ("Save commands")) -> ()
                  }
                }
              }
            }
            n129 = Bundle("Modules 1"="Modules 1", "Modules 2"="Modules 2", "Modules 3"="Modules 3", "Modules 4"="Modules 4", "Modules 5"="Modules 5", "Modules 6"="Modules 6") -> (w89:T7)  [unwired: 1 in]
            n130 = Bundle("Ramp start time (s)"="Ramp start time (s)", "Start freq (MHz)"="Start freq (MHz)", "Sweeps"="Sweeps") -> (w87:T8)  [unwired: 1 in]
            n131 = event shown="[1] \"Tree for programmed measurement\": Double Click" {
              selector: _ -> [_ _]
              dyn-events: _ -> [_ _]
              timeout: 20 -> [_ _]
              event Timeout {
                n132 = event-data() -> ()  [unwired: 1 in, 3 out]
              }
              event "Tree for programmed measurement": Double Click {
                # "Identify which items are double-clicked,  displays dialogs to prompt users enter parameters,and construct command window accordingly"
                n133 = event-data() -> ()  [unwired: 1 in, 10 out]
                n134 = invoke on="Tree for programmed measurement" class="Tree (strict)" method="Double Click"() -> ("Double Click"=w124:string)  [unwired: 3 in, 2 out]
                n135 = case shown="\"Variable loop\"" w124 {
                  frame "False", Default {
                  }
                  frame "Enable module" {
                    n136 = call "Enable module"() -> ("Enable?"=w125:bool, "Module name"=w126:string, "Module index"=w127:dbl, "Module list index"=w128:dbl, "OK"=w129:bool)  [unwired: 14 in, 1 out]
                    n137 = case shown="True" w129 {
                      tunnel: w128 -> [_ w140]
                      tunnel: w127 -> [_ w137]
                      tunnel: w126 -> [_ w134]
                      tunnel: w125 -> [_ w143]
                      frame False {
                      }
                      frame True {
                        w130 = "\n"
                        n138 = local read "Command window"() -> (w145:string)
                        n139 = Number To Decimal String(number=w140) -> (decimal integer string=w139:string)  [unwired: 1 in]
                        n140 = Number To Decimal String(number=w137) -> (decimal integer string=w136:string)  [unwired: 1 in]
                        n141 = case shown="False" w143 {
                          tunnel: ["Disable " ("string") "Enable " ("string")] -> w142
                          frame False {
                          }
                          frame True {
                          }
                        }
                        n142 = Concatenate Strings(" \"" ("string"), w134, "\"" ("string")) -> (w132:string)
                        n143 = Concatenate Strings(w145, w142, "Module list " ("string"), w139, " Module no." ("string"), w136, w132, ", CODE 01" ("string"), w130, w130) -> (w144:string)
                        n144 = local write "Command window"(w144) -> ()
                      }
                    }
                  }
                  frame "Enable MW sweep" {
                    n145 = call "Enable MW sweep"() -> ("Enable?"=w152:bool, "Amplitude"=w148:dbl, "Tau"=w149:dbl, "End frequency"=w150:dbl, "Sweep step index"=w151:dbl, "OK"=w153:bool)  [unwired: 13 in, 1 out]
                    n146 = case shown="True" w153 {
                      tunnel: w152 -> [_ w175]
                      tunnel: w151 -> [_ w174]
                      tunnel: w150 -> [_ w168]
                      tunnel: w149 -> [_ w165]
                      tunnel: w148 -> [_ w159]
                      frame False {
                      }
                      frame True {
                        w154 = "\n"
                        w155 = i16 3 ("precision (6)")
                        n147 = Number To Fractional String(number=w165, precision (6)=w155) -> (F-format string=w162:string)  [unwired: 2 in]
                        n148 = case shown="False" w175 {
                          tunnel: ["Disable " ("string") "Enable " ("string")] -> w176
                          frame False {
                          }
                          frame True {
                          }
                        }
                        n149 = Number To Fractional String(number=w168, precision (6)=w155) -> (F-format string=w167:string)  [unwired: 2 in]
                        n150 = Number To Decimal String(number=w174) -> (decimal integer string=w172:string)  [unwired: 1 in]
                        n151 = local read "Command window"() -> (w177:string)
                        n152 = Concatenate Strings("MW sweep step no." ("string"), w172) -> (w171:string)
                        n153 = Concatenate Strings(": End frequency = " ("string"), w167, " MHz, " ("string")) -> (w166:string)
                        n154 = Number To Fractional String(number=w159, precision (6)=w155) -> (F-format string=w158:string)  [unwired: 2 in]
                        n155 = Concatenate Strings("Tau = " ("string"), w162, ",  " ("string")) -> (w161:string)
                        n156 = Concatenate Strings("Amplitude = " ("string"), w158) -> (w157:string)
                        n157 = Concatenate Strings(w177, w176, w171, w166, w161, w157, ", CODE 02" ("string"), w154, w154) -> (w178:string)
                        n158 = local write "Command window"(w178) -> ()
                      }
                    }
                  }
                  frame "Variable loop" {
                    n159 = call "Variable loop"() -> ("Random?"=w181:bool, "Increment"=w182:dbl, "End value"=w183:dbl, "start value"=w184:dbl, "Variable"=w185:string, "OK"=w186:bool)  [unwired: 13 in, 1 out]
                    n160 = case shown="True" w186 {
                      tunnel: w185 -> [_ w205]
                      tunnel: w184 -> [_ w202]
                      tunnel: w183 -> [_ w194]
                      tunnel: w182 -> [_ w191]
                      tunnel: w181 -> [_ w200]
                      frame False {
                      }
                      frame True {
                        w187 = i16 3 ("precision (6)")
                        w188 = "\n"
                        n161 = local read "Command window"() -> (w190:string)
                        n162 = Number To Fractional String(number=w194, precision (6)=w187) -> (F-format string=w193:string)  [unwired: 2 in]
                        n163 = Number To Fractional String(number=w202, precision (6)=w187) -> (F-format string=w195:string)  [unwired: 2 in]
                        n164 = Number To Fractional String(number=w191, precision (6)=w187) -> (F-format string=w192:string)  [unwired: 2 in]
                        n165 = Select(t=", randomly" ("string"), s=w200, f="" ("string")) -> (s? t:f=w197:string)
                        n166 = Concatenate Strings(w190, "Loop " ("string"), w205, " from " ("string"), w195, " to " ("string"), w193, " with an increment of " ("string"), w192, w197, ", CODE 03" ("string"), w188, w188) -> (w196:string)
                        n167 = local write "Command window"(w196) -> ()
                      }
                    }
                  }
                  frame "End loop" {
                    n168 = disable-structure shown="Disabled" {
                      frame Disabled {
                        n169 = call "End loop"() -> ("variable"=w207:string, "OK"=w208:bool)  [unwired: 17 in, 1 out]
                        n170 = case shown="True" w208 {
                          tunnel: w207 -> [_ w210]
                          frame False {
                          }
                          frame True {
                            w209 = "\n"
                            n171 = local read "Command window"() -> (w214:string)
                            n172 = Concatenate Strings(w214, "End loop " ("string"), w210, ", CODE 04" ("string"), w209, w209) -> (w213:string)
                            n173 = local write "Command window"(w213) -> ()
                          }
                        }
                      }
                      frame Enabled {
                      }
                    }
                  }
                  frame "Run N cycles" {
                    n174 = call "Run N cycles"() -> ("N"=w215:dbl, "OK"=w216:bool)  [unwired: 17 in, 1 out]
                    n175 = case shown="True" w216 {
                      tunnel: w215 -> [_ w221]
                      frame False {
                      }
                      frame True {
                        w217 = "\n"
                        n176 = local read "Command window"() -> (w223:string)
                        n177 = Number To Decimal String(number=w221) -> (decimal integer string=w220:string)  [unwired: 1 in]
                        n178 = Concatenate Strings(w223, "Run experiment for " ("string"), w220, " cycles" ("string"), ", CODE 05" ("string"), w217, w217) -> (w224:string)
                        n179 = local write "Command window"(w224) -> ()
                      }
                    }
                  }
                  frame "Run variable loop" {
                    n180 = call "Run variable loop"() -> ("OK"=w225:bool)  [unwired: 18 in, 1 out]
                    n181 = case shown="True" w225 {
                      frame False {
                      }
                      frame True {
                        w226 = "\n"
                        n182 = local read "Command window"() -> (w230:string)
                        n183 = Concatenate Strings(w230, "Run variable loop" ("string"), ", CODE 06" ("string"), w226, w226) -> (w227:string)
                        n184 = local write "Command window"(w227) -> ()
                      }
                    }
                  }
                  frame "Clear all defined variables" {
                    n185 = call "Clear all defined variables"() -> ("OK"=w231:bool)  [unwired: 18 in, 1 out]
                    n186 = case shown="True" w231 {
                      frame False {
                      }
                      frame True {
                        w232 = "\n"
                        n187 = local read "Command window"() -> (w234:string)
                        n188 = Concatenate Strings(w234, "Clear all defined variables" ("string"), ", CODE 07" ("string"), w232, w232) -> (w233:string)
                        n189 = local write "Command window"(w233) -> ()
                      }
                    }
                  }
                  frame "Config repeat" {
                    n190 = call "Repeat steps"() -> ("Repetition"=w237:dbl, "OK"=w238:bool)  [unwired: 17 in, 1 out]
                    n191 = case shown="True" w238 {
                      tunnel: w237 -> [_ w245]
                      frame False {
                      }
                      frame True {
                        w239 = "\n"
                        n192 = local read "Command window"() -> (w241:string)
                        n193 = Number To Decimal String(number=w245) -> (decimal integer string=w244:string)  [unwired: 1 in]
                        n194 = Concatenate Strings(w241, "Repeat the enclosed steps for " ("string"), w244, " times" ("string"), ", CODE 08" ("string"), w239, w239) -> (w240:string)
                        n195 = local write "Command window"(w240) -> ()
                      }
                    }
                  }
                  frame "Repeat start" {
                    n196 = call "Repeat start"() -> ("OK"=w247:bool)  [unwired: 18 in, 1 out]
                    n197 = case shown="True" w247 {
                      frame False {
                      }
                      frame True {
                        w248 = "\n"
                        n198 = local read "Command window"() -> (w250:string)
                        n199 = Concatenate Strings(w250, "Repeat start" ("string"), ", CODE 09" ("string"), w248, w248) -> (w251:string)
                        n200 = local write "Command window"(w251) -> ()
                      }
                    }
                  }
                  frame "Repeat end" {
                    n201 = call "Repeat end"() -> ("OK"=w253:bool)  [unwired: 18 in, 1 out]
                    n202 = case shown="True" w253 {
                      frame False {
                      }
                      frame True {
                        w254 = "\n"
                        n203 = local read "Command window"() -> (w256:string)
                        n204 = Concatenate Strings(w256, "Repeat end" ("string"), ", CODE 10" ("string"), w254, w254) -> (w257:string)
                        n205 = local write "Command window"(w257) -> ()
                      }
                    }
                  }
                  frame "Move" {
                    n206 = call "Move"() -> ("Movement"=w259:dbl, "Command selected"=w260:dbl, "OK"=w261:bool)  [unwired: 16 in, 1 out]
                    n207 = case shown="True" w261 {
                      tunnel: w260 -> [_ w264]
                      tunnel: w259 -> [_ w265]
                      frame False {
                      }
                      frame True {
                        n208 = Add(x=w264, y=w265) -> (x+y=w266:dbl)
                        n209 = Decrement(x=w264) -> (x-1=w263:dbl)
                        n210 = Decrement(x=w266) -> (x-1=w262:dbl)
                        n211 = stacked-sequence {
                          tunnel: w263 -> [w275 _]
                          tunnel: w262 -> [_ w286]
                          frame #0 {
                            # "Save commands with the command picked deleted"
                            # "if command # smaller than 1, always pick the first command"
                            # "pick command"
                            n212 = local read "Command window"() -> (w274:string)
                            n213 = Concatenate Strings("\n", "\n") -> (w272:string)
                            n214 = for {
                              N: w275 -> [_]
                              shift-right: [w284] -> w273
                              shift-left: w274 -> [w283]
                              tunnel: w272 -> [w282]
                              shift-right: [w279] -> w269
                              shift-left: "" -> [w278]
                              n215 = Match Pattern(string=w283, regular expression=w282) -> (before substring=w281:string, match substring=w280:string, after substring=w284:string)  [unwired: 1 in, 1 out]
                              n216 = Concatenate Strings(w278, w281, w280) -> (w279:string)
                            }
                            n217 = Match Pattern(string=w273, regular expression=w272) -> (before substring=→"temp command":string, after substring=w268:string)  [unwired: 1 in, 2 out]
                            n218 = Concatenate Strings(w269, w268) -> (w267:string)
                            n219 = local write "Command window"(w267) -> ()
                          }
                          frame #1 {
                            # "check if picked \ncommand valid"
                            n220 = local read "temp command"() -> (w285:string)
                            n221 = Equal?(x=w285, y="") -> (x = y?=w287:bool)
                            n222 = case shown="False" w287 {
                              tunnel: w286 -> [w294 _]
                              tunnel: w285 -> [w293 _]
                              frame False {
                                # "check if command is \ngoing to the very front"
                                n223 = local read "Command window"() -> (w291:string)
                                n224 = Decrement(x=w294) -> (x-1=w289:dbl)
                                n225 = Greater?(x=w294, y=0.0) -> (0:w290:bool)
                                n226 = case shown="True" w290 {
                                tunnel: w291 -> [w296 w301]
                                tunnel: w289 -> [_ w304]
                                tunnel: w293 -> [w297 w300]
                                frame False {
                                w298 = "\n"
                                n227 = Concatenate Strings(w297, w298, w298, w296) -> (w295:string)
                                n228 = local write "Command window"(w295) -> ()
                                }
                                frame True {
                                # "check if command is \ngoing to the very end"
                                n229 = Concatenate Strings("\n", "\n") -> (w299:string)
                                n230 = for {
                                N: w304 -> [_]
                                shift-right: [w324] -> w305
                                shift-left: w301 -> [w323]
                                tunnel: w299 -> [w322]
                                n231 = Match Pattern(string=w323, regular expression=w322) -> (after substring=w324:string)  [unwired: 1 in, 3 out]
                                }
                                n232 = Match Pattern(string=w305, regular expression=w299) -> (before substring=w302:string)  [unwired: 1 in, 3 out]
                                n233 = Equal?(x=w302, y="") -> (x = y?=w303:bool)
                                n234 = case shown="True" w303 {
                                tunnel: w302 -> [w317 _]
                                tunnel: w301 -> [w315 w321]
                                tunnel: w300 -> [w312 w320]
                                tunnel: w299 -> [w311 w318]
                                frame False {
                                # "insert picked\ncommand"
                                n235 = Concatenate Strings(w317, w311) -> (w316:string)
                                n236 = Match Pattern(string=w315, regular expression=w316) -> (before substring=w314:string, match substring=w313:string, after substring=w310:string)  [unwired: 1 in, 1 out]
                                n237 = Concatenate Strings(w314, w313, w312, w311, w310) -> (w309:string)
                                n238 = local write "Command window"(w309) -> ()
                                }
                                frame True {
                                n239 = Concatenate Strings(w321, w320, w318) -> (w319:string)
                                n240 = local write "Command window"(w319) -> ()
                                }
                                }
                                }
                                }
                              }
                              frame True {
                              }
                            }
                          }
                        }
                      }
                    }
                  }
                  frame "Swap" {
                    # "swap index A and B\nif index A is not smaller\nthan index B"
                    n241 = call "Swap"() -> ("Command B"=w327:dbl, "Command A"=w328:dbl, "OK"=w332:bool)  [unwired: 16 in, 1 out]
                    n242 = Less?(x=w328, y=w327) -> (x < y?=w331:bool)
                    n243 = case shown="True" w331 {
                      tunnel: w328 -> [w335 w338]
                      tunnel: w327 -> [w336 w337]
                      tunnel: [w336 w338] -> w330
                      tunnel: [w335 w337] -> w329
                      frame False {
                      }
                      frame True {
                      }
                    }
                    n244 = Not Equal?(x=w328, y=w327) -> (x != y?=w334:bool)
                    n245 = Greater Than 0?(x=w327) -> (x > 0?=w325:bool)
                    n246 = Greater Than 0?(x=w328) -> (x > 0?=w326:bool)
                    n247 = Compound Arithmetic op=AND(w326, w325, w332, w334) -> (w333:bool)
                    n248 = case shown="True" w333 {
                      tunnel: w330 -> [_ w353]
                      tunnel: w329 -> [_ w352]
                      frame False {
                      }
                      frame True {
                        w344 = ""
                        n249 = local read "Command window"() -> (w346:string)
                        n250 = Subtract(x=w352, y=w353) -> (x-y=w354:dbl)
                        n251 = Decrement(x=w353) -> (x-1=w356:dbl)
                        n252 = Decrement(x=w354) -> (x-1=w351:dbl)
                        n253 = Concatenate Strings("\n", "\n") -> (w349:string)
                        n254 = for {
                          N: w356 -> [_]
                          shift-right: [w376] -> w355
                          shift-left: w346 -> [w375]
                          tunnel: w349 -> [w374]
                          n255 = Match Pattern(string=w375, regular expression=w374) -> (after substring=w376:string)  [unwired: 1 in, 3 out]
                        }
                        n256 = Match Pattern(string=w355, regular expression=w349) -> (before substring=w340:string, match substring=w348:string, after substring=w345:string)  [unwired: 1 in, 1 out]
                        n257 = for {
                          N: w351 -> [_]
                          shift-right: [w373] -> w350
                          shift-left: w345 -> [w372]
                          tunnel: w349 -> [w371]
                          n258 = Match Pattern(string=w372, regular expression=w371) -> (after substring=w373:string)  [unwired: 1 in, 3 out]
                        }
                        n259 = Match Pattern(string=w350, regular expression=w349) -> (before substring=w339:string, match substring=w347:string)  [unwired: 1 in, 2 out]
                        n260 = Not Equal?(x=w340, y=w344) -> (x != y?=w342:bool)
                        n261 = Not Equal?(x=w344, y=w339) -> (x != y?=w341:bool)
                        n262 = And(x=w342, y=w341) -> (x .and. y?=w343:bool)
                        n263 = case shown="True" w343 {
                          tunnel: w340 -> [_ w370]
                          tunnel: w348 -> [_ w369]
                          tunnel: w339 -> [_ w368]
                          tunnel: w347 -> [_ w367]
                          tunnel: w346 -> [_ w366]
                          tunnel: w345 -> [_ w365]
                          frame False {
                          }
                          frame True {
                            n264 = Concatenate Strings(w370, w369) -> (w361:string)
                            n265 = Concatenate Strings(w368, w367) -> (w363:string)
                            n266 = Match Pattern(string=w366, regular expression=w361) -> (before substring=w364:string)  [unwired: 1 in, 3 out]
                            n267 = Match Pattern(string=w365, regular expression=w363) -> (before substring=w362:string, after substring=w360:string)  [unwired: 1 in, 2 out]
                            n268 = Concatenate Strings(w364, w363, w362, w361, w360) -> (w359:string)
                            n269 = local write "Command window"(w359) -> ()
                          }
                        }
                      }
                    }
                  }
                  frame "Delete" {
                    # "check if index valid"
                    n270 = call "Delete"() -> ("Delete all ?"=w380:bool, "Command selected"=w377:dbl, "OK"=w381:bool)  [unwired: 16 in, 1 out]
                    n271 = Greater Or Equal?(x=w377, y=1.0) -> (x >= y?=w378:bool)
                    n272 = case shown="True" w381 {
                      tunnel: w380 -> [_ w384]
                      tunnel: w378 -> [_ w383]
                      tunnel: w377 -> [_ w382]
                      frame False {
                      }
                      frame True {
                        n273 = case shown="False" w384 {
                          tunnel: w383 -> [w386 _]
                          tunnel: w382 -> [w385 _]
                          frame False {
                            n274 = case shown="True" w386 {
                              tunnel: w385 -> [_ w388]
                              frame False {
                              }
                              frame True {
                                # "delete picked command"
                                # "check if index valid"
                                n275 = local read "Command window"() -> (w387:string)
                                n276 = Decrement(x=w388) -> (x-1=w389:dbl)
                                n277 = Concatenate Strings("\n", "\n") -> (w392:string)
                                n278 = for {
                                N: w389 -> [_]
                                shift-right: [w406] -> w396
                                shift-left: w387 -> [w405]
                                tunnel: w392 -> [w404]
                                # "pick command"
                                n279 = Match Pattern(string=w405, regular expression=w404) -> (after substring=w406:string)  [unwired: 1 in, 3 out]
                                }
                                n280 = Match Pattern(string=w396, regular expression=w392) -> (before substring=w390:string)  [unwired: 1 in, 3 out]
                                n281 = Equal?(x=w390, y="") -> (x = y?=w391:bool)
                                n282 = case shown="False" w391 {
                                tunnel: w390 -> [w399 _]
                                tunnel: w387 -> [w397 _]
                                frame False {
                                w400 = "\n"
                                n283 = Concatenate Strings(w399, w400, w400) -> (w403:string)
                                n284 = Match Pattern(string=w397, regular expression=w403) -> (before substring=w402:string, after substring=w401:string)  [unwired: 1 in, 2 out]
                                n285 = Concatenate Strings(w402, w401) -> (w398:string)
                                n286 = local write "Command window"(w398) -> ()
                                }
                                frame True {
                                }
                                }
                              }
                            }
                          }
                          frame True {
                            # "delete all, empty command window"
                            n287 = local write "Command window"("") -> ()
                          }
                        }
                      }
                    }
                  }
                  frame "Break+Update+Loop" {
                    n288 = call "Break+Update+Loop"() -> ("OK"=w408:bool)  [unwired: 18 in, 1 out]
                    n289 = case shown="True" w408 {
                      frame False {
                      }
                      frame True {
                        w411 = "\n"
                        n290 = local read "Command window"() -> (w410:string)
                        n291 = Concatenate Strings(w410, "Break, update, loop DAC manager" ("string"), ", CODE 11" ("string"), w411, w411) -> (w409:string)
                        n292 = local write "Command window"(w409) -> ()
                      }
                    }
                  }
                  frame "Set DAC manager values" {
                    n293 = call "Set DAC manager values"() -> ("Tau"=w414:string, "Transition"=w415:dbl, "Voltage"=w416:string, "Time"=w417:string, "Step #"=w418:dbl, "Channel"=w419:dbl, "OK"=w420:bool)  [unwired: 12 in, 1 out]
                    n294 = case shown="True" w420 {
                      tunnel: w419 -> [_ w444]
                      tunnel: w418 -> [_ w443]
                      tunnel: w417 -> [_ w437]
                      tunnel: w416 -> [_ w435]
                      tunnel: w415 -> [_ w434]
                      tunnel: w414 -> [_ w430]
                      frame False {
                      }
                      frame True {
                        w421 = "\n"
                        n295 = case shown="3" w434 {
                          tunnel: ["step" ("string") "ramp" ("string") "exp" ("string") "bin" ("string")] -> w432
                          frame 0, Default {
                          }
                          frame 1 {
                          }
                          frame 2 {
                          }
                          frame 3 {
                          }
                        }
                        n296 = Number To Decimal String(number=w444) -> (decimal integer string=w441:string)  [unwired: 1 in]
                        n297 = Number To Decimal String(number=w443) -> (decimal integer string=w439:string)  [unwired: 1 in]
                        n298 = Concatenate Strings("Set DAC manager Channel " ("string"), w441) -> (w429:string)
                        n299 = Concatenate Strings(", Step " ("string"), w439) -> (w428:string)
                        n300 = Concatenate Strings("time: " ("string"), w437) -> (w426:string)
                        n301 = Concatenate Strings(", voltage: " ("string"), w435) -> (w425:string)
                        n302 = Concatenate Strings(", transition: " ("string"), w432) -> (w424:string)
                        n303 = Concatenate Strings(", tau: " ("string"), w430) -> (w423:string)
                        n304 = local read "Command window"() -> (w445:string)
                        n305 = Concatenate Strings(w445, w429, w428, " with the following values: " ("string"), w426, w425, w424, w423, ", CODE 12" ("string"), w421, w421) -> (w446:string)
                        n306 = local write "Command window"(w446) -> ()
                      }
                    }
                  }
                }
              }
            }
            n307 = case shown="True" "Force DAC outputs" {
              frame False {
              }
              frame True {
                n308 = local read "DAC force enables 1"() -> (w467:bool[])
                n309 = local read "DAC force volts 1"() -> (w465:dbl[])
                n310 = local read "DAC force enables 2"() -> (w466:bool[])
                n311 = local read "DAC force volts 2"() -> (w463:dbl[])
                n312 = local read "DAC force enables 3"() -> (w456:bool[])
                n313 = local read "DAC force volts 3"() -> (w454:dbl[])
                n314 = global read "RIO and DAC defaults global.vi" "Static DAC device # 2"() -> (w458:i16)
                n315 = global read "RIO and DAC defaults global.vi" "Static DAC device # 3"() -> (w457:i16)
                n316 = Boolean To (0,1)(Boolean=w467) -> (0, 1=w464:i16[])
                n317 = Boolean To (0,1)(Boolean=w466) -> (0, 1=w462:i16[])
                n318 = Boolean To (0,1)(Boolean=w456) -> (0, 1=w455:i16[])
                n319 = global read "RIO and DAC defaults global.vi" "Static DAC device #"() -> (w459:i16)
                n320 = for {
                  tunnel: w465 -> [w476] mode=indexing
                  tunnel: w464 -> [w475] mode=indexing
                  tunnel: w463 -> [w474] mode=indexing
                  tunnel: w462 -> [w473] mode=indexing
                  tunnel: [w472] -> w460 mode=indexing
                  tunnel: [w471] -> w461 mode=indexing
                  tunnel: w455 -> [w470] mode=indexing
                  tunnel: w454 -> [w469] mode=indexing
                  tunnel: [w468] -> w453 mode=indexing
                  n321 = Multiply(x=w475, y=w476) -> (x*y=w472:dbl)
                  n322 = Multiply(x=w470, y=w469) -> (x*y=w468:dbl)
                  n323 = Multiply(x=w473, y=w474) -> (x*y=w471:dbl)
                }
                n324 = call "AO update.vi"("device"=w459, "data"=w460) -> ()  [unwired: 3 in]
                n325 = call "AO update.vi"("device"=w458, "data"=w461) -> ()  [unwired: 3 in]
                n326 = call "AO update.vi"("device"=w457, "data"=w453) -> ()  [unwired: 3 in]
              }
            }
            n327 = call "GPIB write rf ramp linear up for SG380.vi"("calculate"=TRUE, "do it!"=FALSE, "debug"=FALSE, "time step (ms)"=50.0, "Sweeps"="Sweeps", "start freq (MHz)"="Start freq (MHz)", "start time (sec)"="Ramp start time (s)") -> ("start time 2"=w80:dbl, "calc'd time"=w55:dbl)  [unwired: 2 out]
            "Calc'd time" <- w55
            n328 = Bundle(w89, "Durations"="Durations", w87) -> (w88:T9)  [unwired: 1 in]
            n329 = Select(t=w55, s="Do Evap", f=w80) -> (s? t:f=w79:dbl)
            n330 = case shown="True" "Sequence\nDo write/read" {
              tunnel: w88 -> [_ w528]
              frame False {
                # "Pass"
              }
              frame True {
                # "Write/Read module sequence"
                n331 = stacked-sequence {
                  tunnel: w528 -> [_ w547 _]
                  frame #0 {
                    n332 = property on="Sequence\nDo write/read" class="Bool (strict)"("Value"=FALSE ("Open module"), "DisabledEnum"=T6."Disabled and Grayed Out" ("Disabled")) -> ()  [unwired: 2 in, 2 out]
                  }
                  frame #1 {
                    n333 = call "Save read.vi"("Saveit cluster 1"=w547, "Load from backup"="Load backup?", "Write"="Write/read\nmodule sequence", "Select File"="Select module sequence") -> ("Saveit cluster 2"=w543:T10)
                    n334 = Unbundle(w543) -> (w542:T11, w535:string[], "evap cluster"=w534:T12)
                    n335 = Unbundle(w534) -> ("Start Freq (MHz)"=w533:string, "Ramp Start Time (s)"=w532:string, "Sweeps"=w531:T13)
                    n336 = local write "Ramp start time (s)"(w533) -> ()
                    n337 = local write "Sweeps"(w531) -> ()
                    n338 = local write "Start freq (MHz)"(w532) -> ()
                    n339 = Unbundle(w542) -> ("Module List 1"=w541:T14, "Module List 2"=w540:T14, "Module List 3"=w539:T14, "Module List 4"=w538:T14, "Module List 5"=w537:T14, "Module List 6"=w536:T14)
                    n340 = local write "Modules 1"(w541) -> ()
                    n341 = local write "Modules 2"(w540) -> ()
                    n342 = local write "Modules 3"(w539) -> ()
                    n343 = local write "Modules 4"(w538) -> ()
                    n344 = local write "Modules 5"(w537) -> ()
                    n345 = local write "Modules 6"(w536) -> ()
                    n346 = local write "Durations"(w535) -> ()
                  }
                  frame #2 {
                    w548 = FALSE ("Write/read\nmodule sequence")
                    n347 = local write "Write/read\nmodule sequence"(w548) -> ()
                    n348 = local write "Load backup?"(w548) -> ()
                    n349 = property on="Sequence\nDo write/read" class="Bool (strict)"("DisabledEnum"=T6."Enabled" ("Disabled")) -> ()  [unwired: 2 in, 2 out]
                  }
                }
              }
            }
            n350 = expression code="x*1000"(w79) -> (w54:dbl)
            n351 = global write "Global variables.vi" "Evasp calc'd time"(w54) -> ()
            n352 = Format Value(format string="%10.3f", value (0)=w54) -> (output string=w76:string)  [unwired: 1 in]
            n353 = Replace Array Subset(array="Durations", new element=w76, index=2) -> (w75:string[])
            n354 = local write "Durations"(w75) -> ()
            n355 = case shown="False" "RIO defaults" {
              frame False {
              }
              frame True {
                # "Default RIO"
                n356 = stacked-sequence {
                  frame #0 {
                    n357 = Wait (ms)(milliseconds to wait=u32 100) -> ()  [unwired: 1 out]
                  }
                  frame #1 {
                    n358 = local write "RIO defaults"(FALSE ("RIO defaults")) -> ()
                  }
                  frame #2 {
                    n359 = global read "RIO and DAC defaults global.vi" "Port A default outputs"() -> (w507:bool[])
                    n360 = global read "RIO and DAC defaults global.vi" "Port B default outputs"() -> (w506:bool[])
                    n361 = global read "RIO and DAC defaults global.vi" "Port C default outputs"() -> (w505:bool[])
                    n362 = global read "RIO and DAC defaults global.vi" "Port D default outputs"() -> (w504:bool[])
                    n363 = local write "Port A forced outputs"(w507) -> ()
                    n364 = local write "Port B forced outputs"(w506) -> ()
                    n365 = local write "Port C forced outputs"(w505) -> ()
                    n366 = local write "Port D forced outputs"(w504) -> ()
                  }
                }
              }
            }
            n367 = case shown="True" "Modules\nDo write/read" {
              frame False {
                # "Pass"
              }
              frame True {
                # "Write/Read modules"
                n368 = stacked-sequence {
                  frame #0 {
                    n369 = global write "Modules global.vi" "Error message"("" ("Error message")) -> ()
                    n370 = Not(x="Write/read modules") -> (.not. x?=w520:bool)
                    n371 = global write "Modules global.vi" "Do Write/Read"(TRUE ("Do Write/Read")) -> ()
                    n372 = global write "Modules global.vi" "Read/Write"(w520) -> ()
                    n373 = global write "Modules global.vi" "filename"("Modules save file name") -> ()
                    n374 = property on="Modules\nDo write/read" class="Bool (strict)"("DisabledEnum"=T6."Disabled and Grayed Out" ("Disabled")) -> ()  [unwired: 2 in, 2 out]
                  }
                  frame #1 {
                    n375 = call "read write modules.vi"() -> ()  [unwired: 1 in]
                  }
                  frame #2 {
                    w525 = FALSE ("Do Write/Read")
                    n376 = global read "Modules global.vi" "Error message"() -> (→"Error message":string)
                    n377 = property on="Modules\nDo write/read" class="Bool (strict)"("DisabledEnum"=T6."Enabled" ("Disabled")) -> ()  [unwired: 2 in, 2 out]
                    n378 = local write "Write/read modules"(w525) -> ()
                    n379 = local write "Modules\nDo write/read"(w525) -> ()
                    n380 = global write "Modules global.vi" "Use backup file"(w525) -> ()
                    n381 = global write "Modules global.vi" "Do Write/Read"(w525) -> ()
                  }
                }
              }
            }
            n382 = case shown="False" "Check timing?" {
              tunnel: [w116 3] -> w58
              tunnel: "Run single shot" -> [w117 _]
              tunnel: "Run programmed\ndata acquisition" -> [w115 _]
              frame False {
                n383 = case shown="False" w117 {
                  tunnel: [w118 1] -> w116
                  tunnel: w115 -> [w119 _]
                  frame False {
                    n384 = case shown="False" w119 {
                      tunnel: [0 2] -> w118
                      frame False {
                      }
                      frame True {
                      }
                    }
                  }
                  frame True {
                  }
                }
              }
              frame True {
              }
            }
            n385 = case shown="True" "Clear Error" {
              tunnel: w53 -> [w108 w110]
              tunnel: [w108 w109] -> w52
              frame False {
              }
              frame True {
                n386 = stacked-sequence {
                  tunnel: w110 -> [_ _ w114]
                  tunnel: [_ _ w113] -> w109
                  frame #0 {
                    n387 = Wait (ms)(milliseconds to wait=u32 100) -> ()  [unwired: 1 out]
                  }
                  frame #1 {
                    n388 = local write "Clear Error"(FALSE ("Clear Error")) -> ()
                  }
                  frame #2 {
                    n389 = call <vilib>:"Clear Errors.vi"("error in (no error)"=w114) -> ("error out"=w113:errorcluster)  [unwired: 5 in, 1 out]
                  }
                }
              }
            }
            n390 = case shown="True" "Force RIO outputs" {
              tunnel: "Port A forced outputs" -> [_ w501]
              tunnel: "Port B forced outputs" -> [_ w500]
              tunnel: "Port C forced outputs" -> [_ w499]
              tunnel: "Port D forced outputs" -> [_ w498]
              tunnel: w63 -> [_ w497]
              tunnel: w52 -> [w477 w496]
              tunnel: [w477 w495] -> w62
              frame False {
              }
              frame True {
                n391 = Boolean Array To Number(Boolean array=w501) -> (number=w484:u32)
                n392 = Boolean Array To Number(Boolean array=w500) -> (number=w485:u32)
                n393 = Boolean Array To Number(Boolean array=w499) -> (number=w486:u32)
                n394 = Boolean Array To Number(Boolean array=w498) -> (number=w487:u32)
                n395 = Join Numbers(hi=w485, lo=w484) -> ((hi.lo)=w481:u64)
                n396 = Join Numbers(hi=w487, lo=w486) -> ((hi.lo)=w480:u64)
                n397 = Initialize Array(w480, 1 ("dimension size")) -> (w478:u64[])
                n398 = Initialize Array(w481, 1 ("dimension size")) -> (w479:u64[])
                n399 = call "DIO reset.vi"("error in"=w496, "FPGA VI Reference In"=w497) -> ("error out"=w492:errorcluster, "FPGA VI Reference Out"=w494:refnum<k20>)  [unwired: 8 in]
                n400 = Initialize Array(u64 1 ("element"), u16 1 ("dimension size")) -> (w488:u64[])
                n401 = call "DIO write.vi"("FPGA VI Reference In"=w494, "Timing data"=w488, "Outputs of port A and B"=w479, "Outputs of port C and D"=w478, "error in"=w492) -> ("FPGA VI Reference Out"=w493:refnum<k20>, "error out"=w491:errorcluster)  [unwired: 9 in]
                n402 = call "DIO run.vi"("FPGA VI Reference In"=w493, "error in"=w491) -> ("error out"=w495:errorcluster)  [unwired: 11 in, 6 out]
              }
            }
          }
          frame 1 {
            # "Run single shot"
            n403 = flat-sequence {
              tunnel: w554 -> [w580]
              tunnel: [w579] -> w552
              tunnel: w553 -> [w576]
              tunnel: w556 -> [w577]
              frame #0 {
                w558 = FALSE ("Variable loop enabled")
                n404 = local write "Run programmed\ndata acquisition"(w558) -> ()
                n405 = global write "Global variables.vi" "Variable loop enabled"(w558) -> ()
                n406 = local write "Run single shot"(w558) -> ()
              }
              frame #1 {
                n407 = disable-structure shown="Disabled" {
                  frame Disabled {
                    n408 = call "GPIB write rf ramp linear up for SG380.vi"() -> ()  [unwired: 7 in, 4 out]
                    n409 = call "Send GPIB commands.vi"() -> ()  [unwired: 4 in]
                    n410 = call "Static DAQ prog.vi"() -> ()  [unwired: 4 in]
                    n411 = call "DIO initialize.vi"() -> ()  [unwired: 10 in, 2 out]
                    n412 = call "DIO reset.vi"() -> ()  [unwired: 10 in, 2 out]
                    n413 = call "DIO write.vi"() -> ()  [unwired: 14 in, 2 out]
                    n414 = call "DIO run.vi"() -> ()  [unwired: 13 in, 7 out]
                  }
                  frame Enabled {
                  }
                }
                n415 = global read "RIO and DAC defaults global.vi" "DAC default volts 1"() -> (w568:dbl[])
                n416 = global read "RIO and DAC defaults global.vi" "DAC default volts 2"() -> (w569:dbl[])
                n417 = global read "RIO and DAC defaults global.vi" "DAC default volts 3"() -> (w567:dbl[])
                n418 = local read "Modules 1"() -> (w575:T4)
                n419 = local read "Modules 2"() -> (w572:T4)
                n420 = local read "Modules 3"() -> (w571:T4)
                n421 = local read "Modules 4"() -> (w570:T4)
                n422 = local read "Modules 5"() -> (w573:T4)
                n423 = local read "Modules 6"() -> (w574:T4)
                n424 = local read "Durations"() -> (w563:string[])
                n425 = call "Generate mechine code.vi"("DAC default volts 3"=w567, "Modules 1"=w575, "Modules 2"=w572, "Modules 3"=w571, "Modules 4"=w570, "Modules 5"=w573, "Modules 6"=w574, "DAC default volts 2"=w569, "Section enables"="Section enables", "DAC default volts 1"=w568, "Durations"=w563) -> ("Timing data"=w562:u64[], "Outputs of port A and B"=w566:u64[], "Outputs of port C and D"=w565:u64[], "max module time"=w585:dbl, "AO3"=w561:dbl[][], "AO2"=w560:dbl[][], "AO1"=w559:dbl[][], "Before evap time"=w586:dbl, "GPIB output"=w589:T1)  [unwired: 5 in, 3 out]
                "Max module time" <- w585
                "DO timing indicator" <- w562
                "DO port A/B indicator" <- w566
                "DO port C/D indicator" <- w565
                n426 = local read "Do Evap"() -> (w583:bool)
                n427 = local read "Ramp start time (s)"() -> (w588:string)
                n428 = local read "Start freq (MHz)"() -> (w587:string)
                n429 = local read "Sweeps"() -> (w584:T5)
                n430 = call "DIO write.vi"("FPGA VI Reference In"=w577, "Timing data"=w562, "Outputs of port A and B"=w566, "Outputs of port C and D"=w565, "error in"=w576) -> ("FPGA VI Reference Out"=w591:refnum<k20>, "error out"=w590:errorcluster)  [unwired: 9 in]
                n431 = global read "RIO and DAC defaults global.vi" "Static DAC device #"() -> (w582:i16)
                n432 = global read "RIO and DAC defaults global.vi" "Static DAC device # 2"() -> (w581:i16)
                n433 = global read "RIO and DAC defaults global.vi" "Static DAC device # 3"() -> (w578:i16)
                n434 = stacked-sequence {
                  seq-local: [w602 _ _ _ _ _ _] -> [_ w609 w621 w627 w641 w656 _]
                  seq-local: [w598 _ _ _ _ _ _] -> [_ _ _ _ _ w652 _]
                  seq-local: [w594 _ _ _ _ _ _] -> [_ _ _ _ _ w650 _]
                  seq-local: [w593 _ _ _ _ _ _] -> [_ _ _ _ _ w651 _]
                  tunnel: w591 -> [_ w607 _ _ _ _ _]
                  tunnel: w590 -> [_ w606 _ _ _ _ _]
                  tunnel: w589 -> [_ _ w616 _ w635 _ _]
                  tunnel: w588 -> [_ _ _ w632 _ _ _]
                  tunnel: w587 -> [_ _ _ w631 _ _ _]
                  tunnel: w586 -> [_ _ w617 _ w646 _ _]
                  tunnel: w585 -> [_ _ _ _ w636 _ _]
                  tunnel: w584 -> [_ _ _ w633 _ _ _]
                  tunnel: w583 -> [_ _ _ w624 w648 _ _]
                  tunnel: w559 -> [w600 _ _ _ _ _ _]
                  tunnel: w560 -> [w596 _ _ _ _ _ _]
                  tunnel: w582 -> [w599 _ _ _ _ _ _]
                  tunnel: w581 -> [w597 _ _ _ _ _ _]
                  tunnel: w580 -> [_ w612 _ _ _ _ _]
                  tunnel: [_ w605 _ _ _ _ _] -> w579
                  tunnel: w578 -> [w595 _ _ _ _ _ _]
                  tunnel: w561 -> [w592 _ _ _ _ _ _]
                  frame #0 {
                    w604 = T6."Disabled and Grayed Out" ("Disabled")
                    n435 = property on="Run single shot" class="Bool (strict)"("DisabledEnum"=w604) -> ()  [unwired: 2 in, 2 out]
                    n436 = property on="Run programmed\ndata acquisition" class="Bool (strict)"("DisabledEnum"=w604) -> ()  [unwired: 2 in, 2 out]
                    n437 = call "Static DAQ prog.vi"("device"=w599, "Voltage Array"=w600) -> ("task out"=w598:refnum<k21>)  [unwired: 2 in]
                    n438 = Tick Count (ms)() -> (millisecond timer value=w602:u32)
                    n439 = call "Static DAQ prog.vi"("device"=w597, "Voltage Array"=w596) -> ("task out"=w594:refnum<k21>)  [unwired: 2 in]
                    n440 = local write "Good to go"(FALSE ("Good to go")) -> ()
                    n441 = call "Static DAQ prog.vi"("device"=w595, "Voltage Array"=w592) -> ("task out"=w593:refnum<k21>)  [unwired: 2 in]
                    "AO indicator 1" <- w600
                    "AO indicator 2" <- w596
                    "Boolean" <- TRUE ("Boolean")
                    "AO indicator 3" <- w592
                  }
                  frame #1 {
                    # "measure time from hitting run expt button to the DIO\ntrigger"
                    n442 = Get Date/Time In Seconds() -> (seconds since 1Jan1904=w615:timestamp)
                    n443 = To Double Precision Float(number=w615) -> (double precision float=w614:dbl)
                    "t_start" <- w614
                    n444 = Subtract(x=w614, y=w612) -> (x-y=→"time 2":dbl)
                    n445 = call "DIO run 2.vi"("FPGA VI Reference In"=w607, "error in"=w606) -> ("error out"=w605:errorcluster)  [unwired: 16 in, 1 out]
                    n446 = Tick Count (ms)() -> (millisecond timer value=w610:u32)
                    n447 = Subtract(x=w610, y=w609) -> (x-y=→"millisecond timer value 2":u32)
                    "Boolean 2" <- TRUE ("Boolean 2")
                  }
                  frame #2 {
                    # "do GPIB commands before evap"
                    n448 = call "GPIB write expt GPIB.vi"("Command list 1"=w616, "End time"=w617, "Abs start time"=0.0, "do it!"=TRUE) -> ()
                    n449 = Tick Count (ms)() -> (millisecond timer value=w623:u32)
                    n450 = Subtract(x=w623, y=w621) -> (x-y=→"millisecond timer value 3":u32)
                    "Boolean 3" <- TRUE ("Boolean 3")
                    "GPIB output" <- w616
                  }
                  frame #3 {
                    # "do RF evaporation"
                    n451 = Tick Count (ms)() -> (millisecond timer value=w628:u32)
                    n452 = call "GPIB write rf ramp linear up for SG380.vi"("calculate"=FALSE, "do it!"=w624, "time step (ms)"=50.0, "Sweeps"=w633, "start freq (MHz)"=w631, "start time (sec)"=w632) -> ("timing check"=→"timing check":dbl)  [unwired: 1 in, 3 out]
                    n453 = Subtract(x=w628, y=w627) -> (x-y=→"millisecond timer value 4":u32)
                    "Boolean 4" <- TRUE ("Boolean 4")
                  }
                  frame #4 {
                    n454 = local read "timing check"() -> (w645:dbl)
                    n455 = Multiply(x=w645, y=1000.0) -> (x*y=w643:dbl)
                    n456 = Tick Count (ms)() -> (millisecond timer value=w642:u32)
                    n457 = Add(x=w643, y=w646) -> (x+y=w647:dbl)
                    n458 = Select(t=w647, s=w648, f=w646) -> (s? t:f=w637:dbl)
                    "number 2" <- w637
                    n459 = Subtract(x=w642, y=w641) -> (x-y=→"millisecond timer value 5":u32)
                    n460 = call "GPIB write expt GPIB.vi"("Command list 1"=w635, "End time"=w636, "Abs start time"=w637, "do it!"=TRUE) -> ()
                    "Boolean 5" <- TRUE ("Boolean 5")
                    "number" <- w646
                  }
                  frame #5 {
                    w657 = T6."Enabled" ("Disabled")
                    n461 = local write "Good to go"(TRUE ("Good to go")) -> ()
                    n462 = Wait (ms)(milliseconds to wait=u32 100) -> ()  [unwired: 1 out]
                    n463 = Tick Count (ms)() -> (millisecond timer value=w655:u32)
                    n464 = property on="Run programmed\ndata acquisition" class="Bool (strict)"("DisabledEnum"=w657) -> ()  [unwired: 2 in, 2 out]
                    n465 = property on="Run single shot" class="Bool (strict)"("DisabledEnum"=w657) -> ()  [unwired: 2 in, 2 out]
                    n466 = Subtract(x=w655, y=w656) -> (x-y=→"millisecond timer value 6":u32)
                    n467 = call <vilib>:"DAQmx Clear Task.vi"("task in"=w652) -> ()  [unwired: 14 in, 1 out]
                    n468 = call <vilib>:"DAQmx Clear Task.vi"("task in"=w651) -> ()  [unwired: 14 in, 1 out]
                    n469 = call <vilib>:"DAQmx Clear Task.vi"("task in"=w650) -> ()  [unwired: 14 in, 1 out]
                    "Boolean 6" <- TRUE ("Boolean 6")
                  }
                  frame #6 {
                    w659 = FALSE ("Boolean")
                    n470 = local write "Boolean 2"(w659) -> ()
                    n471 = local write "Boolean 3"(w659) -> ()
                    n472 = local write "Boolean 4"(w659) -> ()
                    n473 = local write "Boolean 5"(w659) -> ()
                    n474 = local write "Boolean 6"(w659) -> ()
                    n475 = local write "Boolean"(w659) -> ()
                  }
                }
              }
            }
            n476 = Get Date/Time In Seconds() -> (seconds since 1Jan1904=w555:timestamp)
            n477 = To Double Precision Float(number=w555) -> (double precision float=w554:dbl)
          }
          frame 2 {
            # "repeat stack pointer"
            # "command window pointer"
            # "Programmed data acquisition"
            n478 = local write "Run programmed\ndata acquisition"(FALSE ("Run programmed\ndata acquisition")) -> ()
            n479 = while {
              shift-right: [w671] -> _
              shift-left: 0 -> [w675]
              shift-right: [w672] -> _
              shift-left: 0 -> [w674]
              tunnel: w663 -> [w667]
              tunnel: w662 -> [w669]
              tunnel: [w668] -> w661
              stop <- w685 stop-if-true
              # "Extract parameters from commands and run experiment as indicated"
              # "Identify commands"
              n480 = global read "Global variables.vi" "Repeat stack"() -> (w679:string)
              n481 = local read "Command window"() -> (w681:string)
              n482 = global read "Global variables.vi" "Repeat enabled"() -> (w670:bool)
              n483 = case shown="False" w670 {
                tunnel: w681 -> [w709 _]
                tunnel: [w709 w710] -> w680
                tunnel: w679 -> [_ w710]
                tunnel: w675 -> [w708 _]
                tunnel: w674 -> [_ w711]
                tunnel: [w708 w711] -> w678
                frame False {
                  # "run commands from command window"
                }
                frame True {
                  # "run commands from repeat stack"
                }
              }
              n484 = call "Pre-decoder.vi"("Command window"=w680, "offset in"=w678) -> ("code"=w687:string, "Command picked"=w684:string, "offset out"=w673:i32, "remaining string"=w686:string)  [unwired: 5 in, 1 out]
              "Command picked" <- w684
              n485 = Equal?(x=w686, y="") -> (x = y?=w677:bool)
              n486 = case shown="True" w670 {
                tunnel: w677 -> [w690 w693]
                tunnel: [w690 FALSE] -> w676
                tunnel: w675 -> [_ _]
                tunnel: w674 -> [w688 _]
                tunnel: w673 -> [w689 w695]
                tunnel: [w689 w691] -> w671
                tunnel: [w688 w692] -> w672
                frame False {
                  # "update command window pointer\nleave repeat stack pointer the same"
                }
                frame True {
                  # "Set command window pointer to repeat\nend, update repeat stack pointer"
                  n487 = global read "Global variables.vi" "Repeat end ptr"() -> (w691:i32)
                  n488 = case shown="True" w693 {
                    tunnel: w695 -> [w696 _]
                    tunnel: [w696 0 ("offset out")] -> w692
                    frame False {
                    }
                    frame True {
                      n489 = global read "Global variables.vi" "Repetition count"() -> (w701:i32)
                      n490 = global read "Global variables.vi" "Total repetition"() -> (w698:i32)
                      n491 = Decrement(x=w698) -> (x-1=w697:i32)
                      n492 = Greater Or Equal?(x=w701, y=w697) -> (x >= y?=w700:bool)
                      n493 = case shown="True" w700 {
                        frame False {
                          (unwired) FALSE
                          # "+1 repetition count"
                          n494 = global read "Global variables.vi" "Repetition count"() -> (w703:i32)
                          n495 = Increment(x=w703) -> (x+1=w702:i32)
                          n496 = global write "Global variables.vi" "Repetition count"(w702) -> ()
                        }
                        frame True {
                          # "repeat finishes, defaults globals"
                          n497 = global write "Global variables.vi" "Repeat enabled"(FALSE ("Repeat enabled")) -> ()
                          n498 = global write "Global variables.vi" "Repetition count"(0 ("Repetition count")) -> ()
                          n499 = global write "Global variables.vi" "Total repetition"(0 ("Total repetition")) -> ()
                          n500 = global write "Global variables.vi" "Repeat stack"("") -> ()
                        }
                      }
                    }
                  }
                }
              }
              n501 = Compound Arithmetic op=OR(w676, "Stop Experiment") -> (w685:bool)
              n502 = case shown="\"03\"" w687 {
                tunnel: w684 -> [w728 w756 w839 w885 _ _ w1125 _ _ _ w1175 w1214]
                tunnel: w673 -> [_ _ _ _ _ _ w1127 _ _ _ _ _]
                tunnel: w667 -> [w713 w751 w838 w881 w1004 w1119 w1124 w1161 w1163 w1165 w1178 w1202]
                tunnel: w669 -> [_ _ _ w880 _ _ _ _ _ _ _ _]
                tunnel: [w713 w751 w838 w879 w1004 w1119 w1124 w1161 w1163 w1165 w1178 w1202] -> w668
                frame "02" {
                  w712 = i16 3 ("precision (6)")
                  # "Enable MW sweep"
                  n503 = call <vilib>:"Trim Whitespace.vi"("string"=w728) -> ("trimmed string"=w730:string)  [unwired: 1 in]
                  n504 = Match Pattern(string=w730, regular expression=" ") -> (before substring=w726:string, after substring=w727:string)  [unwired: 1 in, 2 out]
                  n505 = Scan From String(format string="MW sweep step no.%d: End frequency = %f MHz, Tau = %f, Amplitude = %f ", input string=w727) -> (output 1=w723:i32, output 2=w721:dbl, output 3=w720:dbl, output 4=w719:dbl)  [unwired: 6 in, 3 out]
                  n506 = local read "Sweeps"() -> (w724:T5)
                  n507 = Number To Fractional String(number=w721, precision (6)=w712) -> (F-format string=w718:string)  [unwired: 2 in]
                  n508 = Number To Fractional String(number=w720, precision (6)=w712) -> (F-format string=w717:string)  [unwired: 2 in]
                  n509 = Number To Fractional String(number=w719, precision (6)=w712) -> (F-format string=w716:string)  [unwired: 2 in]
                  n510 = case shown="\"Disable\", Default" w726 {
                    tunnel: [FALSE TRUE] -> w722
                    frame "Disable", Default {
                    }
                    frame "Enable" {
                    }
                  }
                  n511 = Decrement(x=w723) -> (x-1=w714:i32)
                  n512 = in-place {
                    in-place-border: w722 -> [w735]
                    in-place-border: w718 -> [w734]
                    in-place-border: w717 -> [w733]
                    in-place-border: w716 -> [w732]
                    n513 = in-place-array #1(w724, w714) -> (w736:T15)
                    n514 = in-place {
                      in-place-border: w735 -> [w740]
                      in-place-border: w734 -> [w739]
                      in-place-border: w733 -> [w738]
                      in-place-border: w732 -> [w737]
                      n515 = in-place-cluster #2(w736) -> ()  [unwired: 4 out]
                      n516 = in-place-cluster #2("Enable MW"=w740, "MW End freq"=w739, "MW Tau (s)"=w738, "MW Amplitude (dB)"=w737) -> (w731:T15)
                    }
                    n517 = in-place-array #1(w731) -> (w715:T5)  [unwired: 1 out]
                  }
                  n518 = local write "Sweeps"(w715) -> ()
                }
                frame "03" {
                  # "Variable loop"
                  n519 = call <vilib>:"Trim Whitespace.vi"("string"=w756) -> ("trimmed string"=w755:string)  [unwired: 1 in]
                  n520 = Scan From String(format string="Loop %s from %f to %f with an increment of %f", input string=w755) -> (remaining string=w752:string, output 1=w753:string, output 2=w750:dbl, output 3=w749:dbl, output 4=w748:dbl)  [unwired: 6 in, 2 out]
                  n521 = Less Or Equal To 0?(x=w748) -> (x <= 0?=w744:bool)
                  n522 = Not A Number/Path/Refnum?(number/path/refnum=w750) -> (NaN/Path/Refnum?=w747:bool)
                  n523 = Not A Number/Path/Refnum?(number/path/refnum=w749) -> (NaN/Path/Refnum?=w746:bool)
                  n524 = Not A Number/Path/Refnum?(number/path/refnum=w748) -> (NaN/Path/Refnum?=w745:bool)
                  n525 = Compound Arithmetic op=OR(w747, w746, w745, w744) -> (w743:bool)
                  n526 = case shown="False" w743 {
                    tunnel: w753 -> [w769 _]
                    tunnel: w749 -> [w768 _]
                    tunnel: w748 -> [w767 _]
                    tunnel: w750 -> [w766 _]
                    tunnel: w752 -> [w765 _]
                    frame False {
                      n527 = flat-sequence {
                        tunnel: w765 -> [w780]
                        tunnel: w766 -> [w781]
                        tunnel: w767 -> [w782]
                        tunnel: w768 -> [w783]
                        tunnel: w769 -> [w779]
                        tunnel: [w779] -> w764
                        tunnel: [w783] -> w763
                        tunnel: [w782] -> w762
                        tunnel: [w781] -> w761
                        tunnel: [w780] -> w760
                        tunnel: [w772] -> w759
                        tunnel: [w771] -> w758
                        tunnel: [w770] -> w757
                        tunnel: w764 -> [w824]
                        tunnel: w763 -> [w820]
                        tunnel: w762 -> [w819]
                        tunnel: w761 -> [w818]
                        tunnel: w760 -> [w815]
                        tunnel: w759 -> [w806]
                        tunnel: w758 -> [w805]
                        tunnel: w757 -> [w804]
                        frame #0 {
                          # "check if variable exists and ready to overwrite"
                          n528 = global read "Global variables.vi" "indices"() -> (w776:i32[])
                          n529 = global read "Global variables.vi" "Variables defined"() -> (w777:string[])
                          n530 = for {
                            tunnel: w777 -> [w798] mode=indexing
                            tunnel: w779 -> [w799]
                            shift-right: [w797] -> w774
                            shift-left: i32[] [] -> [w795]
                            i -> [w796]
                            n531 = Equal?(x=w798, y=w799) -> (x = y?=w794:bool)
                            n532 = case shown="False" w794 {
                              tunnel: [w800 w803] -> w797
                              tunnel: w796 -> [_ w802]
                              tunnel: w795 -> [w800 w801]
                              frame False {
                              }
                              frame True {
                                n533 = Build Array (concatenate)(w801, w802) -> (w803:i32[])
                              }
                            }
                          }
                          n534 = for {
                            tunnel: w774 -> [w786] mode=indexing
                            tunnel: [w784] -> w773 mode=indexing
                            i -> [w785]
                            n535 = Subtract(x=w786, y=w785) -> (x-y=w784:i32)
                          }
                          n536 = global read "Global variables.vi" "value table"() -> (w775:dbl[][])
                          n537 = for {
                            shift-right: [w792] -> w770
                            shift-left: w777 -> [w793]
                            shift-right: [w788] -> w772
                            shift-left: w776 -> [w791]
                            shift-right: [w787] -> w771
                            shift-left: w775 -> [w790]
                            tunnel: w773 -> [w789] mode=indexing
                            n538 = Delete From Array(array=w790, index (row)=w789) -> (array with subset deleted=w787:dbl[][])  [unwired: 2 in, 1 out]
                            n539 = Delete From Array(array=w791, index=w789) -> (array with subset deleted=w788:i32[])  [unwired: 1 in, 1 out]
                            n540 = Delete From Array(array=w793, index=w789) -> (array with subset deleted=w792:string[])  [unwired: 1 in, 1 out]
                          }
                        }
                        frame #1 {
                          n541 = Initialize Array(0.0 ("element"), 0 ("dimension size")) -> (w821:dbl[])
                          n542 = while {
                            tunnel: w820 -> [w828]
                            tunnel: w819 -> [w829]
                            tunnel: w818 -> [w831]
                            shift-right: [w833] -> w816
                            shift-left: w821 -> [w834]
                            i -> [w837]
                            stop <- w835 stop-if-true
                            n543 = Multiply(x=w829, y=w837) -> (x*y=w836:dbl)
                            n544 = Add(x=w831, y=w836) -> (x+y=w832:dbl)
                            n545 = Build Array (concatenate)(w834, w832) -> (w833:dbl[])
                            n546 = Subtract(x=w828, y=w829) -> (x-y=w830:dbl)
                            n547 = Greater?(x=w832, y=w830) -> (0:w835:bool)
                          }
                          n548 = Build Array (concatenate)(w804, w824) -> (w823:string[])
                          n549 = global write "Global variables.vi" "Variables defined"(w823) -> ()
                          n550 = Match Pattern(string=w815, regular expression="randomly") -> (offset past match=w813:i32)  [unwired: 1 in, 3 out]
                          n551 = Not Equal?(x=w813, y=-1) -> (x != y?=w811:bool)
                          n552 = case shown="False" w811 {
                            tunnel: w816 -> [w825 w827]
                            tunnel: [w825 w826] -> w810
                            frame False {
                            }
                            frame True {
                              n553 = call "Shuffle 1D Array.vim"("array"=w827) -> ("shuffled array"=w826:dbl[])  [unwired: 4 in]
                            }
                          }
                          n554 = Build Array (concatenate)(w806, 0) -> (w807:i32[])
                          n555 = Build Array (concatenate)(w805, w810) -> (w809:dbl[][])
                          n556 = global write "Global variables.vi" "indices"(w807) -> ()
                          n557 = global write "Global variables.vi" "value table"(w809) -> ()
                        }
                      }
                    }
                    frame True {
                    }
                  }
                }
                frame "04", Default {
                  n558 = disable-structure shown="Disabled" {
                    disable-tunnel: w839 -> [w853 _]
                    frame Disabled {
                      n559 = call <vilib>:"Trim Whitespace.vi"("string"=w853) -> ("trimmed string"=w854:string)  [unwired: 1 in]
                      n560 = Scan From String(format string="End loop %s ", input string=w854) -> (output 1=w851:string)  [unwired: 3 in, 3 out]
                      n561 = Search/Split String(string=w851, search string/char (-)=",") -> (substring before match=w848:string)  [unwired: 1 in, 2 out]
                      n562 = global read "Global variables.vi" "Variables defined"() -> (w849:string[])
                      n563 = global read "Global variables.vi" "value table"() -> (w847:dbl[][])
                      n564 = global read "Global variables.vi" "indices"() -> (w846:i32[])
                      n565 = for {
                        tunnel: w849 -> [w863] mode=indexing
                        tunnel: w848 -> [w865]
                        tunnel: w847 -> [w862] mode=indexing
                        tunnel: w846 -> [w857] mode=indexing
                        shift-right: [w861] -> w841
                        shift-left: dbl[][] [] -> [w860]
                        shift-right: [w859] -> w840
                        shift-left: string[] [] -> [w858]
                        shift-right: [w856] -> w842
                        shift-left: i32[] [] -> [w855]
                        n566 = Equal?(x=w863, y=w865) -> (x = y?=w864:bool)
                        n567 = case shown="False" w864 {
                          tunnel: w863 -> [w874 _]
                          tunnel: w862 -> [w873 _]
                          tunnel: [w872 w876] -> w861
                          tunnel: w860 -> [w871 w876]
                          tunnel: [w870 w877] -> w859
                          tunnel: w858 -> [w869 w877]
                          tunnel: w857 -> [w868 _]
                          tunnel: [w867 w875] -> w856
                          tunnel: w855 -> [w866 w875]
                          frame False {
                            n568 = Build Array (concatenate)(w869, w874) -> (w870:string[])
                            n569 = Build Array (concatenate)(w871, w873) -> (w872:dbl[][])
                            n570 = Build Array (concatenate)(w866, w868) -> (w867:i32[])
                          }
                          frame True {
                          }
                        }
                      }
                      n571 = global write "Global variables.vi" "Variables defined"(w840) -> ()
                      n572 = global write "Global variables.vi" "value table"(w841) -> ()
                      n573 = global write "Global variables.vi" "indices"(w842) -> ()
                    }
                    frame Enabled {
                    }
                  }
                }
                frame "05" {
                  # "N cycle"
                  n574 = call <vilib>:"Trim Whitespace.vi"("string"=w885) -> ("trimmed string"=w886:string)  [unwired: 1 in]
                  n575 = Scan From String(format string="Run experiment for %d cycles", input string=w886) -> (output 1=w883:i32)  [unwired: 3 in, 3 out]
                  n576 = flat-sequence {
                    tunnel: w883 -> [w889]
                    tunnel: [w889] -> w882
                    tunnel: [w887] -> w878
                    tunnel: w882 -> [w895]
                    tunnel: w881 -> [w893]
                    tunnel: w880 -> [w894]
                    tunnel: [w892] -> w879
                    tunnel: w878 -> [w891]
                    frame #0 {
                      # "check if iteration time\nvalid"
                      n577 = global write "Global variables.vi" "Variable loop enabled"(FALSE ("Variable loop enabled")) -> ()
                      n578 = global write "Global variables.vi" "Loop total"(w889) -> ()
                      n579 = Greater Or Equal?(x=w889, y=1) -> (x >= y?=w887:bool)
                    }
                    frame #1 {
                      n580 = while {
                        tunnel: w895 -> [w903]
                        tunnel: w894 -> [w900]
                        tunnel: w893 -> [w899]
                        tunnel: [w898] -> w892
                        tunnel: w891 -> [w896]
                        i -> [w902]
                        stop <- w901 stop-if-true
                        n581 = Increment(x=w902) -> (x+1=w897:i32)
                        n582 = stacked-sequence {
                          tunnel: w903 -> [_ _ w1002]
                          tunnel: w897 -> [_ _ w1003]
                          tunnel: [_ _ w999] -> w901
                          tunnel: w900 -> [_ w924 _]
                          tunnel: w899 -> [_ w923 _]
                          tunnel: [_ w922 _] -> w898
                          tunnel: w896 -> [_ w921 _]
                          frame #0 {
                            # "update durations with evaporation time"
                            n583 = local read "Durations"() -> (w909:string[])
                            n584 = local read "Ramp start time (s)"() -> (w910:string)
                            n585 = local read "Start freq (MHz)"() -> (w911:string)
                            n586 = local read "Sweeps"() -> (w912:T5)
                            n587 = local read "Do Evap"() -> (w907:bool)
                            n588 = call "GPIB write rf ramp linear up for SG380.vi"("calculate"=TRUE, "do it!"=FALSE, "debug"=FALSE, "time step (ms)"=50.0, "Sweeps"=w912, "start freq (MHz)"=w911, "start time (sec)"=w910) -> ("start time 2"=w906:dbl, "calc'd time"=w905:dbl)  [unwired: 2 out]
                            n589 = local write "Calc'd time"(w905) -> ()
                            n590 = Select(t=w905, s=w907, f=w906) -> (s? t:f=w916:dbl)
                            n591 = expression code="x*1000"(w916) -> (w904:dbl)
                            n592 = Format Value(format string="%10.3f", value (0)=w904) -> (output string=w913:string)  [unwired: 1 in]
                            n593 = global write "Global variables.vi" "Evasp calc'd time"(w904) -> ()
                            n594 = Replace Array Subset(array=w909, new element=w913, index=2) -> (w908:string[])
                            n595 = local write "Durations"(w908) -> ()
                          }
                          frame #1 {
                            n596 = case shown="True" w921 {
                              tunnel: w924 -> [_ w941]
                              tunnel: w923 -> [w925 w940]
                              tunnel: [w925 w932] -> w922
                              frame False {
                              }
                              frame True {
                                n597 = global read "RIO and DAC defaults global.vi" "Static DAC device #"() -> (w936:i16)
                                n598 = global read "RIO and DAC defaults global.vi" "Static DAC device # 2"() -> (w935:i16)
                                n599 = global read "RIO and DAC defaults global.vi" "Static DAC device # 3"() -> (w929:i16)
                                n600 = local read "Do Evap"() -> (w934:bool)
                                n601 = local read "Ramp start time (s)"() -> (w944:string)
                                n602 = local read "Start freq (MHz)"() -> (w943:string)
                                n603 = local read "Sweeps"() -> (w942:T5)
                                n604 = local read "Modules 1"() -> (w957:T4)
                                n605 = local read "Modules 2"() -> (w956:T4)
                                n606 = local read "Modules 3"() -> (w955:T4)
                                n607 = local read "Modules 4"() -> (w954:T4)
                                n608 = local read "Modules 5"() -> (w953:T4)
                                n609 = local read "Modules 6"() -> (w952:T4)
                                n610 = local read "Section enables"() -> (w951:bool[])
                                n611 = local read "Durations"() -> (w950:string[])
                                n612 = global read "RIO and DAC defaults global.vi" "DAC default volts 1"() -> (w946:dbl[])
                                n613 = global read "RIO and DAC defaults global.vi" "DAC default volts 2"() -> (w945:dbl[])
                                n614 = global read "RIO and DAC defaults global.vi" "DAC default volts 3"() -> (w931:dbl[])
                                n615 = call "Generate mechine code.vi"("DAC default volts 3"=w931, "Modules 1"=w957, "Modules 2"=w956, "Modules 3"=w955, "Modules 4"=w954, "Modules 5"=w953, "Modules 6"=w952, "DAC default volts 2"=w945, "Section enables"=w951, "DAC default volts 1"=w946, "Durations"=w950) -> ("Timing data"=w949:u64[], "Outputs of port A and B"=w948:u64[], "Outputs of port C and D"=w947:u64[], "max module time"=w930:dbl, "AO3"=w926:dbl[][], "AO2"=w927:dbl[][], "AO1"=w928:dbl[][], "Before evap time"=w937:dbl, "GPIB output"=w933:T1)  [unwired: 5 in, 3 out]
                                n616 = local write "Max module time"(w930) -> ()
                                n617 = call "DIO write.vi"("FPGA VI Reference In"=w941, "Timing data"=w949, "Outputs of port A and B"=w948, "Outputs of port C and D"=w947, "error in"=w940) -> ("FPGA VI Reference Out"=w939:refnum<k20>, "error out"=w938:errorcluster)  [unwired: 9 in]
                                n618 = stacked-sequence {
                                seq-local: [w960 _ _ _ _ _] -> [_ _ _ _ _ w996]
                                seq-local: [w959 _ _ _ _ _] -> [_ _ _ _ _ w995]
                                seq-local: [w958 _ _ _ _ _] -> [_ _ _ _ _ w994]
                                tunnel: w944 -> [_ _ _ w978 _ _]
                                tunnel: w943 -> [_ _ _ w979 _ _]
                                tunnel: w942 -> [_ _ _ w980 _ _]
                                tunnel: w928 -> [w966 _ _ _ _ _]
                                tunnel: w927 -> [w964 _ _ _ _ _]
                                tunnel: w939 -> [_ w969 _ _ _ _]
                                tunnel: w938 -> [_ w970 _ _ _ _]
                                tunnel: w930 -> [_ _ _ _ w985 _]
                                tunnel: w937 -> [_ _ w974 _ w989 _]
                                tunnel: w936 -> [w965 _ _ _ _ _]
                                tunnel: w935 -> [w963 _ _ _ _ _]
                                tunnel: w934 -> [_ _ _ w976 w988 _]
                                tunnel: [_ w971 _ _ _ _] -> w932
                                tunnel: w933 -> [_ _ w975 _ w986 _]
                                tunnel: w926 -> [w962 _ _ _ _ _]
                                tunnel: w929 -> [w961 _ _ _ _ _]
                                frame #0 {
                                w967 = T6."Disabled and Grayed Out" ("Disabled")
                                n619 = local write "Good to go"(FALSE ("Good to go")) -> ()
                                n620 = property on="Run programmed\ndata acquisition" class="Bool (strict)"("DisabledEnum"=w967) -> ()  [unwired: 2 in, 2 out]
                                n621 = property on="Run single shot" class="Bool (strict)"("DisabledEnum"=w967) -> ()  [unwired: 2 in, 2 out]
                                n622 = call "Static DAQ prog.vi"("device"=w965, "Voltage Array"=w966) -> ("task out"=w960:refnum<k21>)  [unwired: 2 in]
                                n623 = call "Static DAQ prog.vi"("device"=w963, "Voltage Array"=w964) -> ("task out"=w959:refnum<k21>)  [unwired: 2 in]
                                n624 = call "Static DAQ prog.vi"("device"=w961, "Voltage Array"=w962) -> ("task out"=w958:refnum<k21>)  [unwired: 2 in]
                                }
                                frame #1 {
                                n625 = call "DIO run 2.vi"("FPGA VI Reference In"=w969, "error in"=w970) -> ("error out"=w971:errorcluster)  [unwired: 16 in, 1 out]
                                }
                                frame #2 {
                                # "do GPIB commands before evap"
                                n626 = call "GPIB write expt GPIB.vi"("Command list 1"=w975, "End time"=w974, "Abs start time"=0.0, "do it!"=TRUE) -> ()
                                }
                                frame #3 {
                                n627 = call "GPIB write rf ramp linear up for SG380.vi"("calculate"=FALSE, "do it!"=w976, "time step (ms)"=50.0, "Sweeps"=w980, "start freq (MHz)"=w979, "start time (sec)"=w978) -> ("timing check"=w977:dbl)  [unwired: 1 in, 3 out]
                                n628 = local write "timing check"(w977) -> ()
                                }
                                frame #4 {
                                n629 = local read "timing check"() -> (w987:dbl)
                                n630 = Multiply(x=w987, y=1000.0) -> (x*y=w990:dbl)
                                n631 = Add(x=w990, y=w989) -> (x+y=w992:dbl)
                                n632 = Select(t=w992, s=w988, f=w989) -> (s? t:f=w984:dbl)
                                n633 = call "GPIB write expt GPIB.vi"("Command list 1"=w986, "End time"=w985, "Abs start time"=w984, "do it!"=TRUE) -> ()
                                }
                                frame #5 {
                                w997 = T6."Enabled" ("Disabled")
                                n634 = local write "Good to go"(TRUE ("Good to go")) -> ()
                                n635 = property on="Run single shot" class="Bool (strict)"("DisabledEnum"=w997) -> ()  [unwired: 2 in, 2 out]
                                n636 = property on="Run programmed\ndata acquisition" class="Bool (strict)"("DisabledEnum"=w997) -> ()  [unwired: 2 in, 2 out]
                                n637 = call <vilib>:"DAQmx Clear Task.vi"("task in"=w996) -> ()  [unwired: 14 in, 1 out]
                                n638 = call <vilib>:"DAQmx Clear Task.vi"("task in"=w995) -> ()  [unwired: 14 in, 1 out]
                                n639 = call <vilib>:"DAQmx Clear Task.vi"("task in"=w994) -> ()  [unwired: 14 in, 1 out]
                                n640 = Wait (ms)(milliseconds to wait=u32 100) -> ()  [unwired: 1 out]
                                }
                                }
                              }
                            }
                          }
                          frame #2 {
                            n641 = local read "Stop Experiment"() -> (w1001:bool)
                            n642 = Less Or Equal?(x=w1002, y=w1003) -> (x <= y?=w1000:bool)
                            n643 = Compound Arithmetic op=OR(w1001, w1000) -> (w999:bool)
                          }
                        }
                        n644 = global write "Global variables.vi" "Loop cnt"(w897) -> ()
                      }
                    }
                  }
                }
                frame "06" {
                  # "Run variable loop"
                  n645 = flat-sequence {
                    tunnel: [w1006] -> w1005
                    tunnel: w1005 -> [w1014]
                    frame #0 {
                      n646 = global read "Global variables.vi" "value table"() -> (w1010:dbl[][])
                      n647 = global read "Global variables.vi" "indices"() -> (w1012:i32[])
                      n648 = global write "Global variables.vi" "Variable loop enabled"(TRUE ("Variable loop enabled")) -> ()
                      n649 = Array Size(array=w1010) -> (size(s)=w1011:i32[])
                      n650 = Multiply(x=w1012, y=0) -> (x*y=w1013:i32[])
                      n651 = Index Array(array=w1011, index=1) -> (element=w1006:i32)
                      n652 = global write "Global variables.vi" "indices"(w1013) -> ()
                      n653 = global write "Global variables.vi" "Loop total"(w1006) -> ()
                    }
                    frame #1 {
                      n654 = while {
                        tunnel: w1014 -> [w1018]
                        i -> [w1017]
                        stop <- w1015 stop-if-true
                        n655 = Increment(x=w1017) -> (x+1=w1016:i32)
                        n656 = stacked-sequence {
                          tunnel: w1018 -> [_ w1038 _]
                          tunnel: w1016 -> [_ _ w1116]
                          tunnel: [_ _ w1114] -> w1015
                          frame #0 {
                            # "update durations with evaporation time"
                            n657 = local read "Durations"() -> (w1030:string[])
                            n658 = local read "Ramp start time (s)"() -> (w1033:string)
                            n659 = local read "Start freq (MHz)"() -> (w1034:string)
                            n660 = local read "Sweeps"() -> (w1035:T5)
                            n661 = local read "Do Evap"() -> (w1031:bool)
                            n662 = call "GPIB write rf ramp linear up for SG380.vi"("calculate"=TRUE, "do it!"=FALSE, "debug"=FALSE, "time step (ms)"=50.0, "Sweeps"=w1035, "start freq (MHz)"=w1034, "start time (sec)"=w1033) -> ("start time 2"=w1032:dbl, "calc'd time"=w1020:dbl)  [unwired: 2 out]
                            n663 = Select(t=w1020, s=w1031, f=w1032) -> (s? t:f=w1027:dbl)
                            n664 = local write "Calc'd time"(w1020) -> ()
                            n665 = expression code="x*1000"(w1027) -> (w1019:dbl)
                            n666 = global write "Global variables.vi" "Evasp calc'd time"(w1019) -> ()
                            n667 = Format Value(format string="%10.3f", value (0)=w1019) -> (output string=w1028:string)  [unwired: 1 in]
                            n668 = Replace Array Subset(array=w1030, new element=w1028, index=2) -> (w1029:string[])
                            n669 = local write "Durations"(w1029) -> ()
                          }
                          frame #1 {
                            n670 = Greater?(x=w1038, y=0) -> (0:w1036:bool)
                            n671 = case shown="True" w1036 {
                              frame False {
                              }
                              frame True {
                                n672 = local read "Modules 1"() -> (w1061:T4)
                                n673 = local read "Modules 2"() -> (w1060:T4)
                                n674 = local read "Modules 3"() -> (w1059:T4)
                                n675 = local read "Modules 4"() -> (w1058:T4)
                                n676 = local read "Modules 5"() -> (w1057:T4)
                                n677 = local read "Modules 6"() -> (w1056:T4)
                                n678 = local read "Section enables"() -> (w1051:bool[])
                                n679 = local read "Durations"() -> (w1052:string[])
                                n680 = global read "RIO and DAC defaults global.vi" "Static DAC device #"() -> (w1050:i16)
                                n681 = global read "RIO and DAC defaults global.vi" "Static DAC device # 2"() -> (w1049:i16)
                                n682 = global read "RIO and DAC defaults global.vi" "Static DAC device # 3"() -> (w1048:i16)
                                n683 = local read "Ramp start time (s)"() -> (w1066:string)
                                n684 = local read "Start freq (MHz)"() -> (w1065:string)
                                n685 = local read "Do Evap"() -> (w1067:bool)
                                n686 = local read "Sweeps"() -> (w1064:T5)
                                n687 = global read "RIO and DAC defaults global.vi" "DAC default volts 1"() -> (w1055:dbl[])
                                n688 = global read "RIO and DAC defaults global.vi" "DAC default volts 2"() -> (w1054:dbl[])
                                n689 = global read "RIO and DAC defaults global.vi" "DAC default volts 3"() -> (w1053:dbl[])
                                n690 = call "Generate mechine code.vi"("DAC default volts 3"=w1053, "Modules 1"=w1061, "Modules 2"=w1060, "Modules 3"=w1059, "Modules 4"=w1058, "Modules 5"=w1057, "Modules 6"=w1056, "DAC default volts 2"=w1054, "Section enables"=w1051, "DAC default volts 1"=w1055, "Durations"=w1052) -> ("Timing data"=w1047:u64[], "Outputs of port A and B"=w1046:u64[], "Outputs of port C and D"=w1045:u64[], "max module time"=w1040:dbl, "AO3"=w1042:dbl[][], "AO2"=w1043:dbl[][], "AO1"=w1044:dbl[][], "Before evap time"=w1041:dbl, "GPIB output"=w1039:T1)  [unwired: 5 in, 3 out]
                                n691 = local write "Max module time"(w1040) -> ()
                                n692 = call "DIO write.vi"("Timing data"=w1047, "Outputs of port A and B"=w1046, "Outputs of port C and D"=w1045) -> ("FPGA VI Reference Out"=w1063:refnum<k20>, "error out"=w1062:errorcluster)  [unwired: 11 in]
                                n693 = stacked-sequence {
                                seq-local: [w1070 _ _ _ _ _] -> [_ _ _ _ _ w1104]
                                seq-local: [w1069 _ _ _ _ _] -> [_ _ _ _ _ w1105]
                                seq-local: [w1068 _ _ _ _ _] -> [_ _ _ _ _ w1106]
                                tunnel: w1044 -> [w1078 _ _ _ _ _]
                                tunnel: w1043 -> [w1077 _ _ _ _ _]
                                tunnel: w1042 -> [w1076 _ _ _ _ _]
                                tunnel: w1050 -> [w1075 _ _ _ _ _]
                                tunnel: w1049 -> [w1074 _ _ _ _ _]
                                tunnel: w1048 -> [w1073 _ _ _ _ _]
                                tunnel: w1067 -> [_ _ _ w1090 w1096 _]
                                tunnel: w1066 -> [_ _ _ w1089 _ _]
                                tunnel: w1065 -> [_ _ _ w1088 _ _]
                                tunnel: w1064 -> [_ _ _ w1087 _ _]
                                tunnel: w1040 -> [_ _ _ _ w1094 _]
                                tunnel: w1063 -> [_ w1081 _ _ _ _]
                                tunnel: w1062 -> [_ w1080 _ _ _ _]
                                tunnel: [_ w1079 _ _ _ _] -> _
                                tunnel: w1041 -> [_ _ w1083 _ w1095 _]
                                tunnel: w1039 -> [_ _ w1082 _ w1093 _]
                                frame #0 {
                                w1071 = T6."Disabled and Grayed Out" ("Disabled")
                                n694 = local write "Good to go"(FALSE ("Good to go")) -> ()
                                n695 = property on="Run single shot" class="Bool (strict)"("DisabledEnum"=w1071) -> ()  [unwired: 2 in, 2 out]
                                n696 = property on="Run programmed\ndata acquisition" class="Bool (strict)"("DisabledEnum"=w1071) -> ()  [unwired: 2 in, 2 out]
                                n697 = call "Static DAQ prog.vi"("device"=w1075, "Voltage Array"=w1078) -> ("task out"=w1070:refnum<k21>)  [unwired: 2 in]
                                n698 = call "Static DAQ prog.vi"("device"=w1074, "Voltage Array"=w1077) -> ("task out"=w1069:refnum<k21>)  [unwired: 2 in]
                                n699 = call "Static DAQ prog.vi"("device"=w1073, "Voltage Array"=w1076) -> ("task out"=w1068:refnum<k21>)  [unwired: 2 in]
                                }
                                frame #1 {
                                n700 = call "DIO run 2.vi"("FPGA VI Reference In"=w1081, "error in"=w1080) -> ("error out"=w1079:errorcluster)  [unwired: 16 in, 1 out]
                                }
                                frame #2 {
                                n701 = call "GPIB write expt GPIB.vi"("Command list 1"=w1082, "End time"=w1083, "Abs start time"=0.0, "do it!"=TRUE) -> ()
                                }
                                frame #3 {
                                n702 = call "GPIB write rf ramp linear up for SG380.vi"("calculate"=FALSE, "do it!"=w1090, "time step (ms)"=50.0, "Sweeps"=w1087, "start freq (MHz)"=w1088, "start time (sec)"=w1089) -> ("timing check"=w1086:dbl)  [unwired: 1 in, 3 out]
                                n703 = local write "timing check"(w1086) -> ()
                                }
                                frame #4 {
                                n704 = local read "timing check"() -> (w1097:dbl)
                                n705 = Multiply(x=w1097, y=1000.0) -> (x*y=w1100:dbl)
                                n706 = Add(x=w1100, y=w1095) -> (x+y=w1102:dbl)
                                n707 = Select(t=w1102, s=w1096, f=w1095) -> (s? t:f=w1099:dbl)
                                n708 = call "GPIB write expt GPIB.vi"("Command list 1"=w1093, "End time"=w1094, "Abs start time"=w1099, "do it!"=TRUE) -> ()
                                }
                                frame #5 {
                                w1103 = T6."Enabled" ("Disabled")
                                n709 = property on="Run single shot" class="Bool (strict)"("DisabledEnum"=w1103) -> ()  [unwired: 2 in, 2 out]
                                n710 = property on="Run programmed\ndata acquisition" class="Bool (strict)"("DisabledEnum"=w1103) -> ()  [unwired: 2 in, 2 out]
                                n711 = call <vilib>:"DAQmx Clear Task.vi"("task in"=w1104) -> ()  [unwired: 14 in, 1 out]
                                n712 = Wait (ms)(milliseconds to wait=u32 100) -> ()  [unwired: 1 out]
                                n713 = call <vilib>:"DAQmx Clear Task.vi"("task in"=w1105) -> ()  [unwired: 14 in, 1 out]
                                n714 = call <vilib>:"DAQmx Clear Task.vi"("task in"=w1106) -> ()  [unwired: 14 in, 1 out]
                                }
                                }
                              }
                            }
                          }
                          frame #2 {
                            n715 = global read "Global variables.vi" "value table"() -> (w1109:dbl[][])
                            n716 = Array Size(array=w1109) -> (size(s)=w1111:i32[])
                            n717 = Index Array(array=w1111, index=1) -> (element=w1108:i32)
                            n718 = local read "Stop Experiment"() -> (w1115:bool)
                            n719 = global read "Global variables.vi" "indices"() -> (w1113:i32[])
                            n720 = Less Or Equal?(x=w1108, y=w1116) -> (x <= y?=w1117:bool)
                            n721 = global write "Global variables.vi" "Loop total"(w1108) -> ()
                            n722 = Increment(x=w1113) -> (x+1=w1112:i32[])
                            n723 = Compound Arithmetic op=OR(w1115, w1117) -> (w1114:bool)
                            n724 = global write "Global variables.vi" "indices"(w1112) -> ()
                          }
                        }
                        n725 = global write "Global variables.vi" "Loop cnt"(w1016) -> ()
                      }
                    }
                    frame #2 {
                      n726 = global write "Global variables.vi" "Variable loop enabled"(FALSE ("Variable loop enabled")) -> ()
                    }
                  }
                }
                frame "07" {
                  # "Clear all defined variables"
                  n727 = global write "Global variables.vi" "Variable loop enabled"(FALSE ("Variable loop enabled")) -> ()
                  n728 = global write "Global variables.vi" "value table"(dbl[][] [] ("value table")) -> ()
                  n729 = global write "Global variables.vi" "indices"(i32[] [] ("indices")) -> ()
                  n730 = global write "Global variables.vi" "Variables defined"(string[] [] ("Variables defined")) -> ()
                }
                frame "08" {
                  # "Configure repetition"
                  n731 = flat-sequence {
                    tunnel: w1127 -> [w1135]
                    tunnel: [w1135] -> w1126
                    tunnel: w1125 -> [w1131]
                    tunnel: w1126 -> [w1138]
                    frame #0 {
                      n732 = call <vilib>:"Trim Whitespace.vi"("string"=w1131) -> ("trimmed string"=w1130:string)  [unwired: 1 in]
                      n733 = Scan From String(format string="Repeat the enclosed steps for %s times ", input string=w1130) -> (output 1=w1133:string)  [unwired: 3 in, 3 out]
                      n734 = Decimal String To Number(string=w1133) -> (number=w1134:i32)  [unwired: 2 in, 1 out]
                      n735 = global write "Global variables.vi" "Repetition count"(0 ("Repetition count")) -> ()
                      n736 = global write "Global variables.vi" "Repeat stack"("" ("Repeat stack")) -> ()
                      n737 = global write "Global variables.vi" "Total repetition"(w1134) -> ()
                    }
                    frame #1 {
                      n738 = while {
                        shift-right: [w1154] -> _
                        shift-left: w1138 -> [w1139]
                        shift-right: [w1146] -> _
                        shift-left: FALSE -> [w1144]
                        tunnel: [w1139] -> w1136
                        stop <- w1149 stop-if-true
                        # "detect the commands enclosed by repeat start (CODE 09) nad repeat end (CODE 10), and store them in the Repeat stack for further use"
                        n739 = local read "Command window"() -> (w1155:string)
                        n740 = call "Pre-decoder.vi"("Command window"=w1155, "offset in"=w1139) -> ("Command picked with code"=w1140:string, "code"=w1147:string, "offset out"=w1154:i32, "remaining string"=w1152:string)  [unwired: 5 in, 1 out]
                        n741 = Equal?(x=w1152, y="") -> (x = y?=w1151:bool)
                        n742 = Equal?(x=w1147, y="10") -> (x = y?=w1142:bool)
                        n743 = Not(x=w1142) -> (.not. x?=w1143:bool)
                        n744 = And(x=w1144, y=w1143) -> (x .and. y?=w1141:bool)
                        n745 = Or(x=w1142, y=w1151) -> (x .or. y?=w1149:bool)
                        n746 = Equal?(x=w1147, y="09") -> (x = y?=w1145:bool)
                        n747 = case shown="True" w1141 {
                          tunnel: w1140 -> [_ w1160]
                          frame False {
                          }
                          frame True {
                            w1157 = "\n"
                            n748 = global read "Global variables.vi" "Repeat stack"() -> (w1159:string)
                            n749 = Concatenate Strings(w1157, w1157) -> (w1156:string)
                            n750 = Concatenate Strings(w1159, w1160, w1156) -> (w1158:string)
                            n751 = global write "Global variables.vi" "Repeat stack"(w1158) -> ()
                          }
                        }
                        n752 = Or(x=w1144, y=w1145) -> (x .or. y?=w1146:bool)
                      }
                      n753 = global write "Global variables.vi" "Repeat end ptr"(w1136) -> ()
                    }
                  }
                }
                frame "09" {
                  n754 = global write "Global variables.vi" "Repeat enabled"(TRUE ("Repeat enabled")) -> ()
                }
                frame "10" {
                  n755 = global write "Global variables.vi" "Repeat enabled"(FALSE ("Repeat enabled")) -> ()
                }
                frame "11" {
                  n756 = global write "Global variables.vi" "DAC manager break+update+loop"(TRUE ("DAC manager break+update+loop")) -> ()
                }
                frame "12" {
                  n757 = call <vilib>:"Trim Whitespace.vi"("string"=w1175) -> ("trimmed string"=w1177:string)  [unwired: 1 in]
                  n758 = Scan From String(format string="Set DAC manager Channel %d, Step %d with the following values: time: %[^,], voltage: %[^,], transition: %[^,], tau: %[^,]", input string=w1177) -> (error out=w1167:errorcluster, output 1=w1170:i32, output 2=w1169:i32, output 3=w1174:string, output 4=w1173:string, output 5=w1171:string, output 6=w1172:string)  [unwired: 8 in, 2 out]
                  n759 = call <vilib>:"Clear Errors.vi"("error in (no error)"=w1167) -> ()  [unwired: 5 in, 2 out]
                  n760 = case shown="\"ramp\"" w1171 {
                    tunnel: [0 1 2 3] -> w1168
                    frame "step", Default {
                    }
                    frame "ramp" {
                    }
                    frame "exp" {
                    }
                    frame "bin" {
                    }
                  }
                  n761 = flat-sequence {
                    tunnel: w1174 -> [w1187]
                    tunnel: w1173 -> [w1186]
                    tunnel: w1172 -> [w1184]
                    tunnel: w1170 -> [w1189]
                    tunnel: w1169 -> [w1188]
                    tunnel: w1168 -> [w1185]
                    frame #0 {
                      n762 = Bundle(w1187, w1186, w1185, w1184) -> (w1183:cluster{string, string, i32, string})  [unwired: 1 in]
                      n763 = global write "Global variables.vi" "DAC manager channel"(w1189) -> ()
                      n764 = global write "Global variables.vi" "DAC manager step"(w1188) -> ()
                      n765 = global write "Global variables.vi" "hinge cluster"(w1183) -> ()
                    }
                    frame #1 {
                      n766 = global write "Global variables.vi" "DAC manager set values"(TRUE ("DAC manager set values")) -> ()
                    }
                  }
                }
                frame "01" {
                  # "Enable module"
                  n767 = call <vilib>:"Trim Whitespace.vi"("string"=w1214) -> ("trimmed string"=w1213:string)  [unwired: 1 in]
                  n768 = Match Pattern(string=w1213, regular expression=" ") -> (before substring=w1211:string, after substring=w1210:string)  [unwired: 1 in, 2 out]
                  n769 = Scan From String(format string="Module list %d Module no.%d %[^,],%s", input string=w1210) -> (output 1=w1208:i32, output 2=w1207:i32, output 3=w1195:string)  [unwired: 7 in, 3 out]
                  n770 = String Subset(string=w1195, offset (0)=1) -> (substring=w1193:string)  [unwired: 1 in]
                  n771 = global read "Modules global.vi" "Modules"() -> (w1198:string[])
                  n772 = Decrement(x=w1207) -> (x-1=w1200:i32)
                  n773 = case shown="5" w1208 {
                    selector: w1208 -> [w1231 w1233 w1235 w1237 w1239 w1241]
                    tunnel: [w1232 w1234 w1236 w1238 w1240 w1242] -> w1201
                    tunnel: [w1231 w1233 w1235 w1237 w1239 w1241] -> w1206
                    frame 2 {
                      n774 = local read "Modules 2"() -> (w1232:T4)
                    }
                    frame 3 {
                      n775 = local read "Modules 3"() -> (w1234:T4)
                    }
                    frame 4 {
                      n776 = local read "Modules 4"() -> (w1236:T4)
                    }
                    frame 5 {
                      n777 = local read "Modules 5"() -> (w1238:T4)
                    }
                    frame 6 {
                      n778 = local read "Modules 6"() -> (w1240:T4)
                    }
                    frame 1, Default {
                      n779 = local read "Modules 1"() -> (w1242:T4)
                    }
                  }
                  n780 = Match Pattern(string=w1193, regular expression="\"") -> (before substring=w1191:string)  [unwired: 1 in, 3 out]
                  n781 = Index Array(array=w1201, index=w1200) -> (element=w1199:T16)
                  n782 = Unbundle(w1199) -> ("module"=w1197:u16)  [unwired: 4 out]
                  n783 = Index Array(array=w1198, index=w1197) -> (element=w1196:string)
                  n784 = Equal?(x=w1191, y=w1196) -> (x = y?=w1205:bool)
                  n785 = case shown="\"Disable\", Default" w1211 {
                    tunnel: [FALSE TRUE] -> w1204
                    frame "Disable", Default {
                    }
                    frame "Enable" {
                    }
                  }
                  n786 = in-place {
                    in-place-border: w1205 -> [w1218]
                    in-place-border: w1204 -> [w1217]
                    n787 = in-place-array #3(w1201, w1200) -> (w1216:T16)
                    n788 = in-place {
                      in-place-border: w1218 -> [w1222]
                      in-place-border: w1217 -> [w1221]
                      n789 = in-place-cluster #4(w1216) -> ("enable"=w1220:bool)
                      n790 = case shown="True" w1222 {
                        tunnel: w1220 -> [w1223 _]
                        tunnel: w1221 -> [_ w1224]
                        tunnel: [w1223 w1224] -> w1219
                        frame False {
                        }
                        frame True {
                        }
                      }
                      n791 = in-place-cluster #4("enable"=w1219) -> (w1215:T16)
                    }
                    n792 = in-place-array #3(w1215) -> (w1203:T4)  [unwired: 1 out]
                  }
                  n793 = case shown="2" w1206 {
                    tunnel: w1203 -> [w1225 w1226 w1227 w1228 w1229 w1230]
                    frame 1, Default {
                      n794 = local write "Modules 1"(w1225) -> ()
                    }
                    frame 2 {
                      n795 = local write "Modules 2"(w1226) -> ()
                    }
                    frame 3 {
                      n796 = local write "Modules 3"(w1227) -> ()
                    }
                    frame 4 {
                      n797 = local write "Modules 4"(w1228) -> ()
                    }
                    frame 5 {
                      n798 = local write "Modules 5"(w1229) -> ()
                    }
                    frame 6 {
                      n799 = local write "Modules 6"(w1230) -> ()
                    }
                  }
                }
              }
            }
          }
          frame 3 {
            w1267 = 0.0 ("X Scale.Range:Minimum")
            # "Check timing"
            n800 = local read "Modules 1"() -> (w1265:T4)
            n801 = local read "Modules 2"() -> (w1264:T4)
            n802 = local read "Modules 3"() -> (w1263:T4)
            n803 = local read "Modules 4"() -> (w1262:T4)
            n804 = local read "Modules 5"() -> (w1261:T4)
            n805 = local read "Modules 6"() -> (w1260:T4)
            n806 = local read "Durations"() -> (w1258:string[])
            n807 = local read "Section enables"() -> (w1259:bool[])
            n808 = local write "Check timing?"(FALSE ("Check timing?")) -> ()
            n809 = global read "RIO and DAC defaults global.vi" "DAC default volts 1"() -> (w1254:dbl[])
            n810 = global read "RIO and DAC defaults global.vi" "DAC default volts 2"() -> (w1253:dbl[])
            n811 = global read "RIO and DAC defaults global.vi" "DAC default volts 3"() -> (w1252:dbl[])
            n812 = call "Generate mechine code.vi"("DAC default volts 3"=w1252, "Modules 1"=w1265, "Modules 2"=w1264, "Modules 3"=w1263, "Modules 4"=w1262, "Modules 5"=w1261, "Modules 6"=w1260, "DAC default volts 2"=w1253, "Section enables"=w1259, "DAC default volts 1"=w1254, "Durations"=w1258) -> ("AO1 times"=w1246:dbl[], "Timing data"=w1257:u64[], "AO2 times"=w1247:dbl[], "Outputs of port A and B"=w1256:u64[], "AO3 times"=w1249:dbl[], "Outputs of port C and D"=w1255:u64[], "max module time"=w1251:dbl, "AO3"=w1250:dbl[][], "AO2"=w1245:dbl[][], "AO1"=w1248:dbl[][])  [unwired: 5 in, 2 out]
            n813 = Build Array(w1257, w1256, w1255) -> (w1280:u64[][])
            n814 = call "DAC timeline.vi"("Plot T/F array"="DAC timeline enables 3", "Static DAC Array"=w1250, "times"=w1249) -> ("Timeline"=→"DAC timelines 3":T2)
            n815 = call "DAC timeline.vi"("Plot T/F array"="DAC timeline enables 2", "Static DAC Array"=w1245, "times"=w1247) -> ("Timeline"=→"DAC timelines 2":T2)
            n816 = call "DAC timeline.vi"("Plot T/F array"="DAC timeline enables 1", "Static DAC Array"=w1248, "times"=w1246) -> ("Timeline"=→"DAC timelines 1":T2)
            n817 = call "DIO timeline.vi"("Plot?"="RIO timeline enables", "Array"=w1280) -> ("Timeline"=→"RIO timelines":cluster{u32[], i32[]}[])
            n818 = Add(x=w1251, y=300.0) -> (x+y=w1266:dbl)
            n819 = property on="RIO timelines" class="XYGraph (strict)"("XScale.Minimum"=w1267, "XScale.Maximum"=w1266) -> ()  [unwired: 2 in, 2 out]
            n820 = property on="DAC timelines 1" class="XYGraph (strict)"("XScale.Minimum"=w1267, "XScale.Maximum"=w1266) -> ()  [unwired: 2 in, 2 out]
            n821 = property on="DAC timelines 2" class="XYGraph (strict)"("XScale.Minimum"=w1267, "XScale.Maximum"=w1266) -> ()  [unwired: 2 in, 2 out]
            n822 = property on="DAC timelines 3" class="XYGraph (strict)"("XScale.Minimum"=w1267, "XScale.Maximum"=w1266) -> ()  [unwired: 2 in, 2 out]
          }
        }
        "FPGA Error" <- w43
      }
    }
  }
